vi "WildBugChilGru.vi"() -> ()   [LabVIEW 2014]
uses:
  <vilib>/Utility/miscctls.llb/LVPointTypeDef.ctl
  <vilib>/Utility/xml.llb/Write to XML File(string).vi
  <vilib>/Platform/browser.llb/Open URL in Default Browser (string).vi
  <vilib>/Instr/_visa.llb/VISA Configure Serial Port (Instr).vi
  <vilib>/Analysis/3filter.llb/IIR Filter (DBL).vi
  <vilib>/gmath/NI_Gmath.lvlib
  <vilib>/Analysis/NI_AALBase.lvlib
  <vilib>/ptbypt/NI_PtbyPt.lvlib
panel:
  in  "Autoskalierung Leistung":bool
  in  "Registerkarte 2":enum32{"Seite 1", "Seite 2"}(tab)
  in  "Autoskalierung AFR":bool
  in  "Resetskalierung AFR":bool
  out "Text Rolle":string="Dyno"
  out "Text Zündung":string="Ignition"
  in  "Resetskalierung Leistung":bool
  out "Engine\n[1/min]":cluster{dbl, dbl}(knob) scale=0.0..14000.0
  out "Untersetzung\nermittelt":bool
  out "Rear Tire\n[km/h]":dbl(knob) scale=0.0..200.0
  out "Leistungs-Graph":cluster{dbl[], dbl[]}[](graph)
  out "Untersetzung":dbl format="%.2f"
  out "Untersetzung-Graph":dbl(graph)=4.054054054054054 caption="Untersetzung"
  out "AFR,EGT-Graph":cluster{dbl[], dbl[]}[](graph)
  out "AFR":dbl min=10.0 max=20.0 format="%.1f"
  out "[°C]":dbl
  out "Y-Koord. Graph-Reset-Button (782)":i32=782
  out "Höhe Leistungs-Graph (646)":u32=646
  out "Strecke [m]":dbl=150.82399680000003
  out "dT":dbl=0.02
  out "Cyclecounter":dbl=574.0
  out "Datum+Zeit":string="24.01.2021 11:37"
  out "n(Pmax)":dbl=8917.488266666665
  out "Pmax":dbl=19.664704640664365
  out "Lauf abgebrochen":bool
  out "Auto-Datei":string
  out "Auto-Gespeichert":bool
  in  "Auto-Pfad":path
  in  "Auto-Speichern":bool
  out "n(Rolle) [1/min]":dbl=2046.0
  in  "Fahrzeugdaten":string
  out "Ergebnis":string
  out "Pmax":string="0,0 PS"
  in  "Drucken":bool
  in  "Speichern":bool
  in  "Start":bool
  in  "Ende":bool
  in  "Spenden":bool
  in  "Registerkarte":T1(tab)=enum."Mode & Recalc"
  in  "ignition [Imp/rev]":dbl=1.0 format="%#.2f"
  in  "Übersetzung ermitteln aus":T2(ring)
  in  "gear ratio [1:]":dbl=4.0 min=0.0001
  in  "tire circumferential  [m]":dbl=1.222 min=0.0001
  in  "duration  [s]":u8=5
  in  "nCrank/nDyno":dbl=4.008 format="%#.2f"
  in  "air temperature [°C]":dbl=23.2 format="%#.1g"
  in  "air pressure [mbar]":dbl=100.34 min=0.0001
  in  "Messung Klimadaten":bool=TRUE
  in  "Filter Zündsignal":bool
  in  "v min [km/h]":u16=40
  in  "moving average Mittelwert":u8=35
  in  "difference quotient":u8=12
  in  "n min [1/min]":u16=5000
  in  "torque loss M1 [Nm] @ n1":dbl min=0.0
  in  "dynospeed of torque loss. n1 [1/min]":u16=1 min=1
  in  "torque loss M0 [Nm] @ n = 0":dbl min=0.0
  in  "incr./rev. dyno  [Inkr/U]":u16=100 min=1
  in  "circum. dyno [m]":dbl=0.942 min=0.0001
  in  "Inertia dyno [kgm²]":dbl=0.164 min=0.0001
  in  "record dyno speed":bool
  in  "Lambda":bool caption="Messung Klimadaten"
  in  "AFR, EGT":bool caption="Messung Klimadaten"
  in  "Title Diagram":string
  in  "Recalc":bool
  in  "Leistung":bool=TRUE caption="Messung Klimadaten"
  in  "Logfiles":bool
  out "Datenspeicher":T3={"Fahrzeugdaten"="§$", "Auto-Pfad"="24.01.2021 11:37|", "Rolle [Inkr/U]"=100, "Rollenumfang [m]"=0.942, "Rollenträgheit [kgm²]"=0.164, "Zündung [Imp/U]"=1.0, "Getriebe [1:]"=4.0, "Reifenumfang [m] "=1.222, "element"=0.0, "Gl. Mittelwert"=35, "Differenzenquotient"=12, "AFR EGT"=0, "dT [s]"=0.02, "Strecke [m]"=150.82399680000003, "Lufttemperatur [°C]"=23.2, "Mv: n1 [1/min]"=1.0, "Luftdruck [mbar]"=100.34, "nRolle"=array[575 elements], "nWelle"=array[575 elements], "AFR"=[15.4, 15.4, 15.4, 15.4, 15.4, 15.4, 15.4, 15.4, 15.4, 15.4, 14.9, 14.9, 14.9, 14.9, 14.9, 14.9, 14.9, 14.9, 14.9, 14.9, 15.0, 15.0, 15.0, 15.0, 15.0, 15.4, 15.4, 15.4, 15.4, 15.4, 15.1, 15.1, 15.1, 15.1, 15.1, 14.9, 14.9, 14.9, 14.9, 14.9, 15.2, 15.2, 15.2, 15.2, 15.2, 15.3, 15.3, 15.3, 15.3, 15.3, 15.3, 15.3, 15.3, 15.3, 15.3, 15.0, 15.0, 15.0, 15.0, 15.0, 14.9, 14.9, 14.9, 14.9, 14.9, 15.2, 15.2, 15.2, 15.2, 15.2, 15.4, 15.4, 15.4, 15.4, 15.4, 14.9, 14.9, 14.9, 14.9, 14.9, 14.9, 14.9, 14.9, 14.9, 14.9, 15.1, 15.1, 15.1, 15.1, 15.1, 15.3, 15.3, 15.3, 15.3, 15.3, 15.2, 15.2, 15.2, 15.2, 15.2, 15.0, 15.0, 15.0, 15.0, 15.0, 15.3, 15.3, 15.3, 15.3, 15.3, 15.1, 15.1, 15.1, 15.1, 15.1, 15.3, 15.3, 15.3, 15.3, 15.3, 15.0, 15.0, 15.0, 15.0, 15.0, 15.0, 15.0, 15.0, 15.0, 15.0, 15.3, 15.3, 15.3, 15.3, 15.3, 15.2, 15.2, 15.2, 15.2, 15.2, 15.2, 15.2, 15.2, 15.2, 15.2, 15.0, 15.0, 15.0, 15.0, 15.0, 15.2, 15.2, 15.2, 15.2, 15.2, 15.4, 15.4, 15.4, 15.4, 15.4, 15.2, 15.2, 15.2, 15.2, 15.2, 15.1, 15.1, 15.1, 15.1, 15.1, 15.3, 15.3, 15.3, 15.3, 15.3, 15.3, 15.3, 15.3, 15.3, 15.3, 14.9, 14.9, 14.9, 14.9, 14.9, 15.3, 15.3, 15.3, 15.3, 15.3, 15.0, 15.0, 15.0, 15.0, 15.0, 15.3, 15.3, 15.3, 15.3, 15.3, 15.3, 15.3, 15.3, 15.3, 15.3, 15.2, 15.2, 15.2, 15.2, 15.2, 15.0, 15.0, 15.0, 15.0, 15.0, 15.0, 15.0, 15.0, 15.0, 15.0, 15.2, 15.2, 15.2, 15.2, 15.2, 15.2, 15.2, 15.2, 15.2, 15.2, 15.4, 15.4, 15.4, 15.4, 15.4, 15.0, 15.0, 15.0, 15.0, 15.0, 15.1, 15.1, 15.1, 15.1, 15.1, 15.0, 15.0, 15.0, 15.0, 15.0, 15.1, 15.1, 15.1, 15.1, 15.1, 15.1, 15.1, 15.1, 15.1, 15.1, 15.4, 15.4, 15.4, 15.4, 15.4, 15.0, 15.0, 15.0, 15.0, 15.0, 15.2, 15.2, 15.2, 15.2, 15.2, 15.0, 15.0, 15.0, 15.0, 15.0, 15.0, 15.0, 15.0, 15.0, 15.0, 15.3, 15.3, 15.3, 15.3, 15.3, 14.9, 14.9, 14.9, 14.9, 14.9, 15.2, 15.2, 15.2, 15.2, 15.2, 15.1, 15.1, 15.1, 15.1, 15.1, 15.2, 15.2, 15.2, 15.2, 15.2, 15.0, 15.0, 15.0, 15.0, 15.0, 15.4, 15.4, 15.4, 15.4, 15.4, 15.0, 15.0, 15.0, 15.0, 15.0, 15.4, 15.4, 15.4, 15.4, 15.4, 15.1, 15.1, 15.1, 15.1, 15.1, 15.3, 15.3, 15.3, 15.3, 15.3, 15.0, 15.0, 15.0, 15.0, 15.0, 14.9, 14.9, 14.9, 14.9, 14.9, 15.1, 15.1, 15.1, 15.1, 15.1, 15.1, 15.1, 15.1, 15.1, 15.1, 15.0, 15.0, 15.0, 15.0, 15.0, 15.2, 15.2, 15.2, 15.2, 15.2, 15.4, 15.4, 15.4, 15.4, 15.4, 15.2, 15.2, 15.2, 15.2, 15.2, 15.2, 15.2, 15.2, 15.2, 15.2, 14.9, 14.9, 14.9, 14.9, 14.9, 15.0, 15.0, 15.0, 15.0, 15.0, 15.2, 15.2, 15.2, 15.2, 15.2, 14.9, 14.9, 14.9, 14.9, 14.9, 15.1, 15.1, 15.1, 15.1, 15.1, 15.2, 15.2, 15.2, 15.2, 15.2, 15.0, 15.0, 15.0, 15.0, 15.0, 15.0, 15.0, 15.0, 15.0, 15.0, 15.2, 15.2, 15.2, 15.2, 15.2, 15.3, 15.3, 15.3, 15.3, 15.3, 15.0, 15.0, 15.0, 15.0, 15.0, 15.0, 15.0, 15.0, 15.0, 15.0, 15.1, 15.1, 15.1, 15.1, 15.1, 15.3, 15.3, 15.3, 15.3, 15.3, 15.1, 15.1, 15.1, 15.1, 15.1, 15.3, 15.3, 15.3, 15.3, 15.3, 15.1, 15.1, 15.1, 15.1, 15.1, 15.0, 15.0, 15.0, 15.0, 15.0, 15.2, 15.2, 15.2, 15.2, 15.2, 14.9, 14.9, 14.9, 14.9, 14.9, 15.3, 15.3, 15.3, 15.3, 15.3, 15.1, 15.1, 15.1, 15.1, 15.1, 15.4, 15.4, 15.4, 15.4, 15.4, 15.4, 15.4, 15.4, 15.4, 15.4, 15.4, 15.4, 15.4, 15.4, 15.4, 14.9, 14.9, 14.9, 14.9, 14.9, 15.2, 15.2, 15.2, 15.2, 15.2, 15.0, 15.0, 15.0, 15.0, 15.0, 15.0, 15.0, 15.0, 15.0, 15.0, 15.4, 15.4, 15.4, 15.4, 15.4, 15.4, 15.4, 15.4, 15.4, 15.4, 15.4, 15.4, 15.4, 15.4, 15.4, 15.1, 15.1, 15.1, 15.1, 15.1, 15.2, 15.2, 15.2, 15.2, 15.2, 15.2, 15.2, 15.2, 15.2, 15.2, 15.1, 15.1, 15.1, 15.1, 15.1, 15.2, 15.2, 15.2, 15.2, 15.2, 15.3, 15.3, 15.3, 15.3, 15.3], "EGT"=array[575 elements], "Übersetzung ermitteln aus"=0, "[s]"=5.0, "Mv: M0 [Nm]"=0.0, "Mv: M1 [Nm]"=0.0, "n vom Gas [1/min]"=5000.0, "dT-Array [s]"=array[575 elements], [], "Boolesch"=TRUE, "Serielle Schnittstelle"="COM6", "nKuWe/nRolle"=4.008, "v vom Gas [km/h]"=40.0}
  out "COM-Fehlerrate":string="0 / 0,0%"
  in  "Konfiguration:":bool
  out "Füllstand Lesepuffer":u64(slide)=1 scale=1.0..100.0
  out "Lesepuffer":string="\r\n"
  in  "Serielle Schnittstelle":refnum<visa-resource-name>="COM6"
  # "Power measurement:\n1. constant speed\n2. START [F1]\n3. hold speed\n4. @ GO: open throttle\n5. release gas"
  # "WildBugGruChil Dyno v3.0.1"
  # "ratio engine/dyno"
  # "manual <> measure"
  # "Dashboard <> Measure"
  # "AFR / l &  EGT"
  # "AFR <> l"
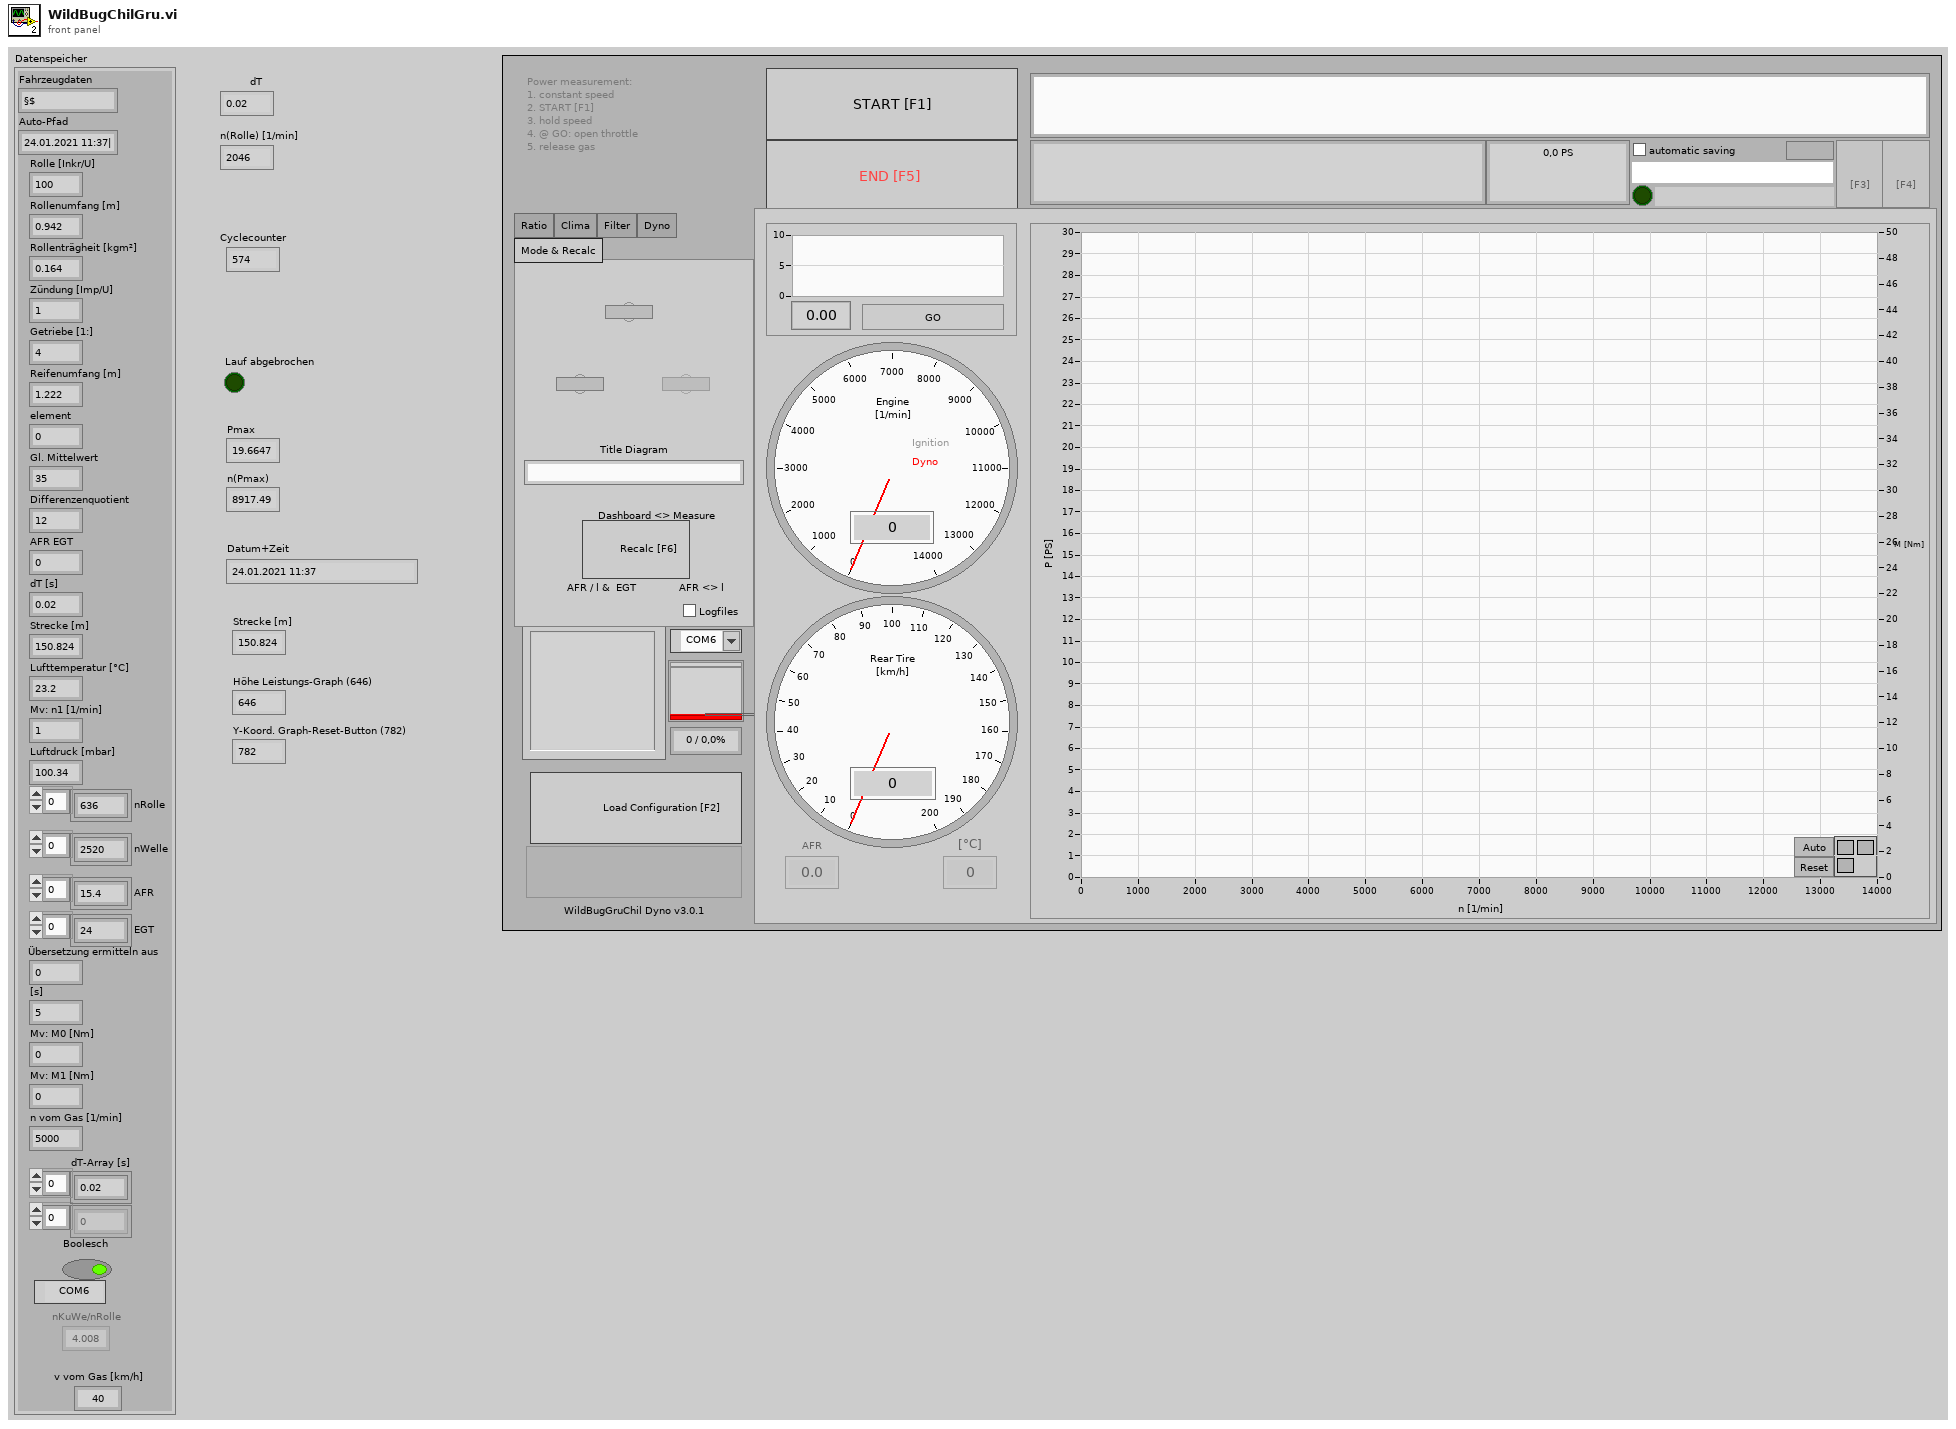
[diagram p1: front panel]
types:
  T1 = enum32{"Ratio", "Clima", "Filter", "Dyno", "Mode & Recalc"}
  T2 = enum8{"ignition signal", "gear ratio & speed", "nCrank / nDyno", "vario (km/h)"}
  T3 = cluster{"Fahrzeugdaten":string, "Auto-Pfad":string, "Rolle [Inkr/U]":u16, "Rollenumfang [m]":dbl, "Rollenträgheit [kgm²]":dbl, "Zündung [Imp/U]":dbl, "Getriebe [1:]":dbl, "Reifenumfang [m] ":dbl, "element":dbl, "Gl. Mittelwert":u8, "Differenzenquotient":u8, "AFR EGT":u8, "dT [s]":dbl, "Strecke [m]":dbl, "Lufttemperatur [°C]":dbl, "Mv: n1 [1/min]":dbl, "Luftdruck [mbar]":dbl, "nRolle":dbl[], "nWelle":dbl[], "AFR":dbl[], "EGT":dbl[], "Übersetzung ermitteln aus":u8, "[s]":dbl, "Mv: M0 [Nm]":dbl, "Mv: M1 [Nm]":dbl, "n vom Gas [1/min]":dbl, "dT-Array [s]":dbl[], i32[], "Boolesch":bool, "Serielle Schnittstelle":refnum<visa-resource-name>, "nKuWe/nRolle":dbl, "v vom Gas [km/h]":dbl}
  T4 = enum8{"Enabled", "Disabled", "Disabled and Grayed Out"}
  T5 = cluster{"Fahrzeugdaten":string, "Auto-Pfad":string, "Rolle [Inkr/U]":u16, "Rollenumfang [m]":dbl, "Rollenträgheit [kgm²]":dbl, "Zündung [Imp/U]":dbl, "Getriebe [1:]":dbl, "Reifenumfang [m] ":dbl, "element":dbl, "Gl. Mittelwert":u8, "Differenzenquotient":u8, u8, "dT [s]":dbl, "Strecke [m]":dbl, "Lufttemperatur [°C]":dbl, "Mv: n1 [1/min]":dbl, "Luftdruck [mbar]":dbl, "nRolle":dbl[], "nWelle":dbl[], "AFR":dbl[], "EGT":dbl[], "Übersetzung ermitteln aus":u8, "[s]":dbl, "Mv: M0 [Nm]":dbl, "Mv: M1 [Nm]":dbl, "n vom Gas [1/min]":dbl, "dT-Array [s]":dbl[], i32[], "Boolesch":bool, "Serielle Schnittstelle":refnum<visa-resource-name>, "nKuWe/nRolle":dbl, "v vom Gas [km/h]":dbl}
  T6 = enum32{"invalid app kind", "Development System", "Run Time System", "Student Edition", "Embedded LabVIEW", "Evaluation", "Custom"}
  T7 = cluster{string, string, "incr./rev. dyno  [Inkr/U]":u16, "circum. dyno [m]":dbl, "Inertia dyno [kgm²]":dbl, "ignition [Imp/rev]":dbl, "gear ratio [1:]":dbl, "tire circumferential  [m] ":dbl, "mean value":dbl, "moving average Mittelwert":u8, "difference quotient ":u8, u32, dbl, "Strecke [m]":dbl, "air temperature [°C]":dbl, "dynospeed of torque loss. n1 [1/min]":u16, "air pressure [mbar]":dbl, dbl[], dbl[], dbl[], dbl[], "Übersetzung ermitteln aus":enum8{"ignition signal", "gear ratio & speed", "nCrank / nDyno", "vario (km/h)"}, "duration  [s]":u8, "torque loss M0 [Nm] @ n = 0 ":dbl, "torque loss M1 [Nm] @ n1":dbl, "n min [1/min]":u16, dbl[], i32[], "Messung Klimadaten":bool, "VISA-Referenz (Ausgang)":refnum<visa-resource-name>, "nCrank/nDyno":dbl, "v min [km/h]":u16}
  T8 = typedef "LVPointTypeDef.ctl" = cluster{"Horizontal":i16, "Vertical":i16}
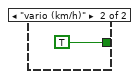
[diagram p3: hidden frame]
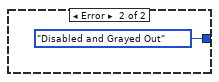
[diagram p5: hidden frame]
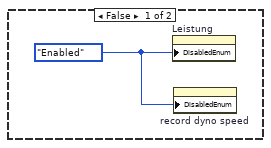
[diagram p6: hidden frame]
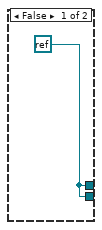
[diagram p7: hidden frame]
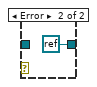
[diagram p8: hidden frame]
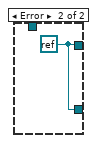
[diagram p9: hidden frame]
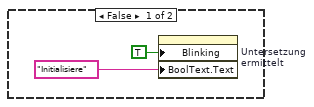
[diagram p10: hidden frame]
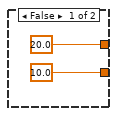
[diagram p11: hidden frame]
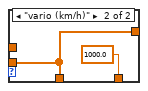
[diagram p20: hidden frame]
diagram:
  w3 = FALSE
  n1 = while {
    stop <- w9 stop-if-true
    n2 = event shown="[6] \"Spenden\": Wertänderung" {
      selector: _ -> [_ _ _ _ _ _ _ _ _ _ _ _ _ _ _ _ _ _]
      dyn-events: _ -> [_ _ _ _ _ _ _ _ _ _ _ _ _ _ _ _ _ _]
      timeout: _ -> [_ _ _ _ _ _ _ _ _ _ _ _ _ _ _ _ _ _]
      tunnel: [_ _ _ TRUE _ _ _ _ _ _ _ _ _ _ _ _ _ _] -> w9
      event "Konfiguration:": Value Change {
        n3 = event-data() -> ("OldVal"=w11:bool)  [unwired: 1 in, 5 out]
        n4 = flat-sequence {
          tunnel: [w55] -> w12
          tunnel: w11 -> [w55]
          tunnel: w12 -> [w56]
          frame #0 {
            n5 = property on="Datenspeicher" class="Cluster (strikt)"() -> ("Value"=w54:T3)  [unwired: 2 in, 2 out]
            n6 = call "LoadCluster (SubVI).vi"("Datenspeicher"=w54) -> ("Value"=w53:T5)  [unwired: 8 in, 2 out]
            n7 = Unbundle(w53) -> ("Fahrzeugdaten"=w20:string, "Auto-Pfad"=w28:string, "Rolle [Inkr/U]"=w52:u16, "Rollenumfang [m]"=w51:dbl, "Rollenträgheit [kgm²]"=w50:dbl, "Zündung [Imp/U]"=w49:dbl, "Getriebe [1:]"=w48:dbl, "Reifenumfang [m]"=w47:dbl, "Gl. Mittelwert"=w46:u8, "Differenzenquotient"=w45:u8, w15:u8, "Lufttemperatur [°C]"=w44:dbl, "Mv: n1 [1/min]"=w25:dbl, "Luftdruck [mbar]"=w43:dbl, "Übersetzung ermitteln aus"=w40:u8, "[s]"=w42:dbl, "Mv: M0 [Nm]"=w36:dbl, "Mv: M1 [Nm]"=w35:dbl, "n vom Gas [1/min]"=w41:dbl, "Boolesch"=w39:bool, "nKuWe/nRolle"=w38:dbl, "v vom Gas [km/h]"=w37:dbl)  [unwired: 10 out]
            n8 = property on="duration  [s]" class="DigWert (strikt)"("Value"=w42) -> ()  [unwired: 2 in, 2 out]
            n9 = property on="Übersetzung ermitteln aus" class="Enum (strikt)"("Val(Sgnl)"=w40) -> ()  [unwired: 2 in, 2 out]
            n10 = property on="incr./rev. dyno  [Inkr/U]" class="DigWert (strikt)"("Value"=w52) -> ()  [unwired: 2 in, 2 out]
            n11 = property on="circum. dyno [m]" class="DigWert (strikt)"("Value"=w51) -> ()  [unwired: 2 in, 2 out]
            n12 = property on="Inertia dyno [kgm²]" class="DigWert (strikt)"("Value"=w50) -> ()  [unwired: 2 in, 2 out]
            n13 = property on="ignition [Imp/rev]" class="DigWert (strikt)"("Value"=w49) -> ()  [unwired: 2 in, 2 out]
            n14 = property on="gear ratio [1:]" class="DigWert (strikt)"("Value"=w48) -> ()  [unwired: 2 in, 2 out]
            n15 = property on="tire circumferential  [m]" class="DigWert (strikt)"("Value"=w47) -> ()  [unwired: 2 in, 2 out]
            n16 = property on="moving average Mittelwert" class="DigWert (strikt)"("Value"=w46) -> ()  [unwired: 2 in, 2 out]
            n17 = property on="difference quotient" class="DigWert (strikt)"("Value"=w45) -> ()  [unwired: 2 in, 2 out]
            n18 = property on="air temperature [°C]" class="DigWert (strikt)"("Value"=w44) -> ()  [unwired: 2 in, 2 out]
            n19 = property on="air pressure [mbar]" class="DigWert (strikt)"("Value"=w43) -> ()  [unwired: 2 in, 2 out]
            n20 = property on="n min [1/min]" class="DigWert (strikt)"("Value"=w41) -> ()  [unwired: 2 in, 2 out]
            n21 = property on="Messung Klimadaten" class="Bool. (strikt)"("Val(Sgnl)"=w39) -> ()  [unwired: 2 in, 2 out]
            n22 = property on="nCrank/nDyno" class="DigWert (strikt)"("Value"=w38) -> ()  [unwired: 2 in, 2 out]
            n23 = property on="v min [km/h]" class="DigWert (strikt)"("Value"=w37) -> ()  [unwired: 2 in, 2 out]
            n24 = Number To Boolean Array(number=w15) -> (Boolean array=w17:bool[])
            n25 = property on="torque loss M1 [Nm] @ n1" class="DigWert (strikt)"("Value"=w35) -> ()  [unwired: 2 in, 2 out]
            n26 = property on="torque loss M0 [Nm] @ n = 0" class="DigWert (strikt)"("Value"=w36) -> ()  [unwired: 2 in, 2 out]
            n27 = Index Array(array=w17, index=0) -> (element=w14:bool)
            n28 = Index Array(array=w17, index=1) -> (element=w13:bool)
            n29 = property on="Lambda" class="Bool. (strikt)"("Val(Sgnl)"=w13) -> ()  [unwired: 2 in, 2 out]
            n30 = property on="AFR, EGT" class="Bool. (strikt)"("Value"=w14) -> ()  [unwired: 2 in, 2 out]
            n31 = Search/Split String "führende Fahrzeugdaten wegschneiden"(string=w20, search string/char (-)="§$") -> (substring before match=w19:string, match + rest of string=w22:string)  [unwired: 1 in, 1 out]
            n32 = Search/Split String "führendes Datum+Zeit wegschneiden"(string=w28, search string/char (-)="|") -> (substring before match=w29:string, match + rest of string=w32:string)  [unwired: 1 in, 1 out]
            n33 = Max & Min(x=1, y=w25) -> (max(x,y)=w27:dbl)  [unwired: 1 out]
            n34 = String Subset(string=w22, offset (0)=2) -> (substring=w21:string)  [unwired: 1 in]
            n35 = String Subset(string=w32, offset (0)=1) -> (substring=w30:string)  [unwired: 1 in]
            n36 = String To Path(string=w30) -> (path=w34:path)
            n37 = property on="dynospeed of torque loss. n1 [1/min]" class="DigWert (strikt)"("Value"=w27) -> ()  [unwired: 2 in, 2 out]
            n38 = property on="Title Diagram" class="Str"("Value"=w21) -> ()  [unwired: 2 in, 2 out]
            n39 = property on="Datum+Zeit" class="Str"("Value"=w29) -> ()  [unwired: 2 in, 2 out]
            n40 = property on="Fahrzeugdaten" class="Str"("Value"=w19) -> ()  [unwired: 2 in, 2 out]
            n41 = property on="Auto-Pfad" class="Pfad"("Value"=w34) -> ()  [unwired: 2 in, 2 out]
          }
          frame #1 {
            n42 = property on="Konfiguration:" class="Bool. (strikt)"("Value"=w56) -> ()  [unwired: 2 in, 2 out]
          }
        }
      }
      event "Drucken": Value Change {
        n43 = event-data() -> ("OldVal"=w57:bool)  [unwired: 1 in, 5 out]
        n44 = flat-sequence {
          tunnel: [w65] -> w58
          tunnel: w57 -> [w65]
          tunnel: w58 -> [w66]
          frame #0 {
            n45 = control-ref of="Fahrzeugdaten"() -> (w63:refnum<vi>)
            n46 = control-ref of="Ergebnis"() -> (w62:refnum<vi>)
            n47 = control-ref of="Title Diagram"() -> (w61:refnum<vi>)
            n48 = control-ref of="Leistungs-Graph"() -> (w64:refnum<vi>)
            n49 = control-ref of="AFR,EGT-Graph"() -> (w60:refnum<vi>)
            n50 = local read "AFR, EGT"() -> (w59:bool)
            n51 = call "PrintGraph (SubVI).vi"("AFR,EGT-Graph Ref"=w60, "AFR, EGT"=w59, "Überschrift"=w61, "Ergebnis"=w62, "Fahrzeugdaten"=w63, "P+M Graph Ref"=w64) -> ()  [unwired: 6 in]
          }
          frame #1 {
            n52 = property on="Drucken" class="Bool. (strikt)"("Value"=w66) -> ()  [unwired: 2 in, 2 out]
          }
        }
      }
      event "Speichern": Value Change {
        n53 = event-data() -> ("OldVal"=w67:bool)  [unwired: 1 in, 5 out]
        n54 = flat-sequence {
          frame #0 {
            n55 = property on="Auto-Gespeichert" class="Bool. (strikt)"("Value"=FALSE) -> ()  [unwired: 2 in, 2 out]
            n56 = property on="Auto-Datei" class="Str"("Value"="") -> ()  [unwired: 2 in, 2 out]
          }
          frame #1 {
            n57 = local read "Auto-Pfad"() -> (w79:path)
            n58 = property on="Auto-Speichern" class="Bool. (strikt)"() -> ("Value"=w73:bool)  [unwired: 2 in, 2 out]
            n59 = call <vilib>:"Check if File or Folder Exists.vi"("path"=w79) -> ("file or folder exists?"=w78:bool, "dup path"=w75:path)  [unwired: 8 in, 1 out]
            n60 = Not(x=w78) -> (.not. x?=w77:bool)
            n61 = And(x=w73, y=w77) -> (x .and. y?=w76:bool)
            n62 = And(x=w73, y=w78) -> (x .and. y?=w70:bool)
            n63 = call "Meldung an Benutzer2"("Enable"=w76) -> ()  [unwired: 9 in, 2 out]
            n64 = case shown="True" w70 {
              tunnel: [path "" w95] -> w80
              tunnel: w75 -> [_ w94]
              tunnel: ["" w88] -> w71
              frame False {
              }
              frame True {
                n65 = Get Date/Time In Seconds() -> (seconds since 1Jan1904=w98:timestamp)
                n66 = local read "Pmax"() -> (w91:dbl)
                n67 = local read "n(Pmax)"() -> (w90:dbl)
                n68 = Path To String(path=w94) -> (string=w97:string)
                n69 = Format Into String(format string="%,; %.1f_%d.xml" ("Format-String"), w91, w90) -> (resulting string=w86:string)  [unwired: 2 in, 1 out]
                n70 = Format Date/Time String(time format string (%c)="%y%m%d_%H%M%S_", seconds (now)=w98) -> (date/time string=w87:string)  [unwired: 1 in]
                n71 = Concatenate Strings(w97, "\\", w87, w86) -> (w96:string)
                n72 = Concatenate Strings(w87, w86) -> (w88:string)
                n73 = String To Path(string=w96) -> (path=w95:path)
              }
            }
            n74 = control-ref of="Datenspeicher"() -> (w81:refnum<vi>)
            n75 = call "SaveCluster (SubVI).vi"("selected path"=w80, "Datenspeicher 2"=w81) -> ("Kein Fehler"=w74:bool)
            n76 = And(x=w70, y=w74) -> (x .and. y?=w72:bool)
            n77 = case shown="True" w72 {
              tunnel: w71 -> [_ w83]
              frame False {
              }
              frame True {
                n78 = property on="Auto-Gespeichert" class="Bool. (strikt)"("Value"=TRUE) -> ()  [unwired: 2 in, 2 out]
                n79 = property on="Auto-Datei" class="Str"("Value"=w83) -> ()  [unwired: 2 in, 2 out]
              }
            }
          }
        }
        n80 = local write "Speichern"(w67) -> ()
      }
      event "Ende": Value Change {
        w108 = 0.0 ("element")
        n81 = event-data() -> ("OldVal"=w106:bool)  [unwired: 1 in, 5 out]
        n82 = local read "Datenspeicher"() -> (w109:T3)
        n83 = flat-sequence {
          tunnel: [w138] -> w105
          tunnel: w106 -> [w138]
          frame #0 {
            n84 = Wait (ms)(milliseconds to wait=u32 200) -> ()  [unwired: 1 out]
          }
        }
        n85 = Unbundle By Name(w109) -> ("Auto-Pfad"=w100:string, "Rolle [Inkr/U]"=w130:u16, "Rollenumfang [m]"=w129:dbl, "Rollenträgheit [kgm²]"=w128:dbl, "Zündung [Imp/U]"=w127:dbl, "Getriebe [1:]"=w126:dbl, "Reifenumfang [m]"=w125:dbl, "Gl. Mittelwert"=w124:u8, "Differenzenquotient"=w123:u8, "Fahrzeugdaten"=w122:string, "Lufttemperatur [°C]"=w121:dbl, "Mv: n1 [1/min]"=w120:dbl, "Luftdruck [mbar]"=w118:dbl, "nRolle"=w119:dbl[], "Übersetzung ermitteln aus"=w117:u8, "[s]"=w116:dbl, "Mv: M0 [Nm]"=w115:dbl, "Mv: M1 [Nm]"=w114:dbl, "n vom Gas [1/min]"=w113:dbl, "Boolesch"=w112:bool, "Serielle Schnittstelle"=w107:refnum<visa-resource-name>, "nWelle"=w104:dbl[], "AFR"=w102:dbl[], "EGT"=w101:dbl[], "v vom Gas [km/h]"=w103:dbl, "AFR EGT"=w99:u8)  [unwired: 3 out]
        n86 = call <vilib>:"Application Directory.vi"() -> ("Application Directory"=w133:path)
        n87 = local write "Ende"(w105) -> ()
        n88 = Bundle By Name(cluster=w109, "Auto-Pfad"=w100, "Rolle [Inkr/U]"=w130, "Rollenumfang [m]"=w129, "Rollenträgheit [kgm²]"=w128, "Zündung [Imp/U]"=w127, "Getriebe [1:]"=w126, "Reifenumfang [m]"=w125, "element"=0.0, "Gl. Mittelwert"=w124, "Differenzenquotient"=w123, "Fahrzeugdaten"=w122, "element"=w108, "element"=w108, "Lufttemperatur [°C]"=w121, "Mv: n1 [1/min]"=w120, "Luftdruck [mbar]"=w118, "nRolle"=w119, "Übersetzung ermitteln aus"=w117, "[s]"=w116, "Mv: M0 [Nm]"=w115, "Mv: M1 [Nm]"=w114, "n vom Gas [1/min]"=w113, "Boolesch"=w112, "Serielle Schnittstelle"=w107, "nWelle"=w104, "AFR"=w102, "EGT"=w101, "v vom Gas [km/h]"=w103, "AFR EGT"=w99) -> (w110:T3)
        n89 = Build Path(base path=w133, name or relative path="Konfig.xml") -> (appended path=w131:path)
        n90 = Flatten To XML(anything=w110) -> (xml string=w135:string)
        n91 = call-poly <vilib>:"Write to XML File.vi"("XML Input"=w135, "XML File Path"=w131) -> ("error out"=w134:errorcluster)  [unwired: 7 in, 2 out]
        n92 = case shown="Kein Fehler" w134 {
          frame No Error {
          }
          frame Error {
          }
        }
      }
      event "Serielle Schnittstelle": Value Change {
        n93 = event-data() -> ()  [unwired: 1 in, 6 out]
        n94 = property on="Start" class="Bool. (strikt)"("DisabledEnum"=T4."Enabled" ("Deaktiviert")) -> ()  [unwired: 2 in, 2 out]
      }
      event "Messung Klimadaten": Value Change {
        n95 = event-data() -> ("NewVal"=w140:bool)  [unwired: 1 in, 5 out]
        n96 = case shown="True" w140 {
          frame True {
            w141 = T4."Disabled and Grayed Out" ("Deaktiviert")
            n97 = property on="air temperature [°C]" class="DigWert (strikt)"("DisabledEnum"=w141) -> ()  [unwired: 2 in, 2 out]
            n98 = property on="air pressure [mbar]" class="DigWert (strikt)"("DisabledEnum"=w141) -> ()  [unwired: 2 in, 2 out]
          }
          frame False {
            w142 = T4."Enabled" ("Deaktiviert")
            n99 = property on="air temperature [°C]" class="DigWert (strikt)"("DisabledEnum"=w142) -> ()  [unwired: 2 in, 2 out]
            n100 = property on="air pressure [mbar]" class="DigWert (strikt)"("DisabledEnum"=w142) -> ()  [unwired: 2 in, 2 out]
          }
        }
      }
      event "Spenden": Value Change {
        n101 = event-data() -> ()  [unwired: 1 in, 6 out]
        n102 = case shown="True" "Spenden" {
          frame False {
          }
          frame True {
            (unwired) "https://www.paypal.com/cgi-bin/webscr?cmd=_s-xclick&hosted_button_id=5HCL4L3EEXS64&source=url"  # Spende an august.gruendl@gmx.at
            w144 = "https://www.paypal.com/cgi-bin/webscr?cmd=_s-xclick&hosted_button_id=8SA7Y5J5P5N3W&source=url"  # Spende an WildBugChilGru@gmx.net
            n103 = call-poly <vilib>:"Open URL in Default Browser.vi"("URL"=w144) -> ()  [unwired: 5 in, 2 out]
          }
        }
      }
      event "Recalc": Value Change {
        n104 = event-data() -> ("OldVal"=w147:bool)  [unwired: 1 in, 5 out]
        n105 = property on="Recalc" class="Bool. (strikt)"("Value"=w147) -> ()  [unwired: 2 in, 2 out]
        n106 = property on="Datenspeicher" class="Cluster (strikt)"() -> ("Value"=w145:T3)  [unwired: 2 in, 2 out]
        n107 = call "ReCalc.vi"("Berechnen"=TRUE, "Datenspeicher"=w145) -> ()  [unwired: 3 in]
      }
      event "Übersetzung ermitteln aus": Value Change {
        w151 = 2
        w157 = 1
        n108 = event-data() -> ("NewVal"=w175:T2)  [unwired: 1 in, 5 out]
        n109 = case shown="\"vario (km/h)\"" w175 {
          tunnel: [w191 w192 w194 w197] -> w176
          tunnel: [w191 w193 w194 w196] -> w173
          tunnel: [w191 w192 w195 w196] -> w165
          tunnel: [w191 w193 w195 w197] -> w172
          tunnel: [T4."Enabled" ("Deaktiviert") w192 w194 w196] -> w171
          frame "vario (km/h)" {
            w191 = T4."Disabled and Grayed Out" ("Deaktiviert")
          }
          frame "nCrank / nDyno" {
            w193 = T4."Enabled" ("Deaktiviert")
            w192 = T4."Disabled and Grayed Out" ("Deaktiviert")
          }
          frame "ignition signal", Default {
            w195 = T4."Enabled" ("Deaktiviert")
            w194 = T4."Disabled and Grayed Out" ("Deaktiviert")
          }
          frame "gear ratio & speed" {
            w196 = T4."Disabled and Grayed Out" ("Deaktiviert")
            w197 = T4."Enabled" ("Deaktiviert")
          }
        }
        n110 = case shown="\"vario (km/h)\"" w175 {
          tunnel: ["n [1/min]" "M [Nm]"] -> w174
          tunnel: [200.0 14000.0] -> w164
          tunnel: ["v [km/h]" "n [1/min]"] -> w149
          tunnel: [14000.0 50.0] -> w170
          tunnel: [u32 16777216 w185] -> w168
          tunnel: [u32 16711680 w185] -> w167
          tunnel: [FALSE TRUE] -> w166
          frame "vario (km/h)" {
          }
          frame Default {
            w185 = u32 9868950
          }
        }
        n111 = property on="Leistungs-Graph" class="XYGraph (strikt)"("ActYScl"=w157, "YScale.NameLbl.Text"=w174, "YScale.Maximum"=w170, "XScale.NameLbl.Text"=w149, "XScale.Maximum"=w164) -> ("Height"=w163:u32, "YScale.NameLbl.Width"=w162:u32, "Top"=w159:i32, "Width"=w154:u32, "XScale.NameLbl.Width"=w153:u32, "Left"=w152:i32)  [unwired: 2 in, 2 out]
        n112 = property on="Text Zündung" class="Str"("Text.TextColor"=w167) -> ()  [unwired: 2 in, 2 out]
        n113 = property on="Welle [1/min]" class="Drehknopf (strikt)"("Active Slider"=1, "FG Color"=w168) -> ()  [unwired: 2 in, 2 out]
        n114 = property on="Text Rolle" class="Str"("Visible"=w166) -> ()  [unwired: 2 in, 2 out]
        n115 = Subtract(x=w154, y=w153) -> (x-y=w155:u32)
        n116 = Subtract(x=w163, y=w162) -> (x-y=w161:u32)
        n117 = Divide(x=w155, y=w151) -> (x/y=w156:dbl)
        n118 = Divide(x=w161, y=w151) -> (x/y=w160:dbl)
        n119 = Add(x=w156, y=w152) -> (x+y=w150:dbl)
        n120 = Add(x=w160, y=w159) -> (x+y=w158:dbl)
        n121 = property on="Leistungs-Graph" class="XYGraph (strikt)"("ActYScl"=w157, "YScale.NameLbl.Top"=w158, "XScale.NameLbl.Left"=w150) -> ()  [unwired: 2 in, 2 out]
        n122 = property on="AFR,EGT-Graph" class="XYGraph (strikt)"("XScale.Maximum"=w164, "XScale.NameLbl.Text"=w149, "XScale.NameLbl.Left"=w150) -> ()  [unwired: 2 in, 2 out]
        n123 = property on="nCrank/nDyno" class="DigWert (strikt)"("DisabledEnum"=w173) -> ()  [unwired: 2 in, 2 out]
        n124 = property on="v min [km/h]" class="DigWert (strikt)"("DisabledEnum"=w171) -> ()  [unwired: 2 in, 2 out]
        n125 = property on="n min [1/min]" class="DigWert (strikt)"("DisabledEnum"=w172) -> ()  [unwired: 2 in, 2 out]
        n126 = property on="gear ratio [1:]" class="DigWert (strikt)"("DisabledEnum"=w176) -> ()  [unwired: 2 in, 2 out]
        n127 = property on="tire circumferential  [m]" class="DigWert (strikt)"("DisabledEnum"=w176) -> ()  [unwired: 2 in, 2 out]
        n128 = property on="ignition [Imp/rev]" class="DigWert (strikt)"("DisabledEnum"=w165) -> ()  [unwired: 2 in, 2 out]
        n129 = property on="duration  [s]" class="DigWert (strikt)"("DisabledEnum"=w165) -> ()  [unwired: 2 in, 2 out]
        n130 = property on="Filter Zündsignal" class="Bool. (strikt)"("DisabledEnum"=w165) -> ()  [unwired: 2 in, 2 out]
        n131 = property on="Leistungs-Graph" class="XYGraph (strikt)"() -> ("Width"=w148:u32)  [unwired: 2 in, 2 out]
        n132 = property on="AFR,EGT-Graph" class="XYGraph (strikt)"("Width"=w148) -> ()  [unwired: 2 in, 2 out]
      }
      event "Resetskalierung Leistung": Value Change {
        w199 = 0.0
        n133 = event-data() -> ()  [unwired: 1 in, 6 out]
        n134 = local read "Übersetzung ermitteln aus"() -> (w202:T2)
        n135 = case shown="\"vario (km/h)\"" w202 {
          tunnel: [14000.0 200.0] -> w200
          tunnel: [50.0 14000.0] -> w201
          frame Default {
          }
          frame "vario (km/h)" {
          }
        }
        n136 = property on="Leistungs-Graph" class="XYGraph (strikt)"("XScale.Maximum"=w200, "XScale.Minimum"=w199, "ActYScl"=w199, "YScale.Maximum"=30.0, "YScale.Minimum"=w199, "ActYScl"=1, "YScale.Maximum"=w201, "YScale.Minimum"=w199) -> ()  [unwired: 2 in, 2 out]
        n137 = property on="AFR,EGT-Graph" class="XYGraph (strikt)"("XScale.Maximum"=w200, "XScale.Minimum"=w199) -> ()  [unwired: 2 in, 2 out]
      }
      event "Auto-Speichern": Value Change {
        n138 = event-data() -> ("NewVal"=w208:bool)  [unwired: 1 in, 5 out]
        n139 = case shown="True" w208 {
          frame False {
          }
          frame True {
            n140 = local read "Auto-Pfad"() -> (w211:path)
            n141 = call <vilib>:"Check if File or Folder Exists.vi"("path"=w211) -> ("file or folder exists?"=w209:bool)  [unwired: 8 in, 2 out]
            n142 = Not(x=w209) -> (.not. x?=w210:bool)
            n143 = call "Meldung an Benutzer"("Enable"=w210) -> ()  [unwired: 9 in, 2 out]
            n144 = local write "Auto-Speichern"(w209) -> ()
          }
        }
      }
      event "Fahrzeugdaten": Value Change {
        # "Fahrzeugdaten auf 3 Zeilen begrenzen\n(Recalc ist nur auf max. 3 Zeilen ausgelegt)"
        n145 = event-data() -> ("OldVal"=w214:string, "NewVal"=w215:string)  [unwired: 1 in, 4 out]
        n146 = Spreadsheet String To Array(delimiter (Tab)="\n", format string="%s", spreadsheet string=w215, array type (2D Dbl)=string[] []) -> (array=w217:string[])
        n147 = Array Size "Zeilenanzahl"(array=w217) -> (size(s)=w216:i32)
        n148 = Greater?(x=w216, y=3) -> (0:w213:bool)
        n149 = case shown="True" w213 {
          tunnel: w214 -> [_ w221]
          frame False {
          }
          frame True {
            n150 = flat-sequence {
              tunnel: w221 -> [w223]
              frame #0 {
                n151 = call "Meldung an Benutzer3"("Enable"=TRUE) -> ()  [unwired: 9 in, 2 out]
              }
              frame #1 {
                n152 = property on="Fahrzeugdaten" class="Str"("Value"=w223) -> ()  [unwired: 2 in, 2 out]
              }
            }
          }
        }
      }
      event "AFR, EGT": Value Change {
        n153 = event-data() -> ("NewVal"=w224:bool)  [unwired: 1 in, 5 out]
        n154 = local read "Y-Koord. Graph-Reset-Button (782)"() -> (w232:i32)
        n155 = local read "Höhe Leistungs-Graph (646)"() -> (w233:u32)
        n156 = control-ref of="Resetskalierung Leistung"() -> (w230:refnum<vi>)
        n157 = control-ref of="Autoskalierung Leistung"() -> (w225:refnum<vi>)
        n158 = control-ref of="AFR,EGT-Graph"() -> (w229:refnum<vi>)
        n159 = control-ref of="Leistungs-Graph"() -> (w231:refnum<vi>)
        n160 = control-ref of="Lambda"() -> (w226:refnum<vi>)
        n161 = property on="Autoskalierung AFR" class="Bool. (strikt)"("Visible"=w224) -> ()  [unwired: 2 in, 2 out]
        n162 = property on="Resetskalierung AFR" class="Bool. (strikt)"("Visible"=w224) -> ()  [unwired: 2 in, 2 out]
        n163 = control-ref of="AFR"() -> (w228:refnum<vi>)
        n164 = control-ref of="[°C]"() -> (w227:refnum<vi>)
        n165 = call "Enable_AFR_EGT_Graph (SubVI).vi"("Leistungsgraph"=w231, "AFR EGT"=w224, "Y-Koord. Graph-Reset-Button (782)"=w232, "Lambda"=w226, "Reset Skalierung"=w230, "Höhe Leistungs-Graph"=w233, "AFR EGT Gaph"=w229, "Auto Skalierung"=w225, "AFR"=w228, "EGT [°C]"=w227, "Skalierungsfaktor Leistungsgraph"=0.6666666666666666) -> ()  [unwired: 5 in]
      }
      event "Lambda": Value Change {
        w240 = 14.7
        w241 = 0.06802721088435375
        w257 = 0
        n166 = event-data() -> ("NewVal"=w242:bool)  [unwired: 1 in, 5 out]
        n167 = case shown="False" w242 {
          tunnel: ["AFR" "l"] -> w267
          tunnel: ["Anwendung" "Symbol"] -> w266
          tunnel: [20.0 1.6] -> w265
          tunnel: [10.0 0.4] -> w269
          tunnel: [w270 w275] -> w268
          tunnel: [w270 w275] -> w236
          frame False {
            w270 = 1
          }
          frame True {
            w275 = 2
          }
        }
        n168 = property on="AFR,EGT-Graph" class="XYGraph (strikt)"("ActYScl"=w257, "YScale.NameLbl.Text"=w267, "YScale.NameLbl.FontName"=w266, "YScale.Maximum"=w265, "YScale.Minimum"=w269, "YScale.Precision"=w268) -> ("Height"=w264:u32, "YScale.NameLbl.Width"=w263:u32, "Top"=w259:i32)  [unwired: 2 in, 2 out]
        n169 = property on="AFR" class="DigWert (strikt)"("Caption.Text"=w267, "Caption.FontName"=w266, "Format"=0, "Precision"=w236) -> ()  [unwired: 2 in, 2 out]
        n170 = Subtract(x=w264, y=w263) -> (x-y=w262:u32)
        n171 = local read "AFR,EGT-Graph"() -> (w253:cluster{dbl[], dbl[]}[])
        n172 = Divide(x=w262, y=2) -> (x/y=w260:dbl)
        n173 = Add(x=w260, y=w259) -> (x+y=w258:dbl)
        n174 = property on="AFR,EGT-Graph" class="XYGraph (strikt)"("ActYScl"=w257, "YScale.NameLbl.Top"=w258, "Active Plot"=0) -> ()  [unwired: 2 in, 2 out]
        n175 = Index Array(array=w253, index=1) -> (element=w245:cluster{dbl[], dbl[]})
        n176 = Index Array(array=w253, index=0) -> (element=w254:cluster{dbl[], dbl[]})
        n177 = local read "AFR"() -> (w239:dbl)
        n178 = Unbundle(w254) -> (w247:dbl[], w250:dbl[])
        n179 = Multiply(x=w241, y=w239) -> (x*y=w238:dbl)
        n180 = Multiply(x=w239, y=w240) -> (x*y=w237:dbl)
        n181 = Multiply(x=w241, y=w250) -> (x*y=w251:dbl[])
        n182 = Multiply(x=w240, y=w250) -> (x*y=w249:dbl[])
        n183 = Select(t=w251, s=w242, f=w249) -> (s? t:f=w248:dbl[])
        n184 = Select(t=w238, s=w242, f=w237) -> (s? t:f=w243:dbl)
        n185 = Bundle(w247, w248) -> (w246:cluster{dbl[], dbl[]})  [unwired: 1 in]
        n186 = local write "AFR"(w243) -> ()
        n187 = Build Array(w246, w245) -> (w244:cluster{dbl[], dbl[]}[])
        n188 = property on="AFR,EGT-Graph" class="XYGraph (strikt)"("Value"=w244) -> ()  [unwired: 2 in, 2 out]
      }
      event "Leistung": Value Change {
        w280 = 0.0
        n189 = event-data() -> ("NewVal"=w283:bool)  [unwired: 1 in, 5 out]
        n190 = case shown="True" w283 {
          tunnel: [w285 w288] -> w284
          tunnel: [w285 w289] -> w282
          frame False {
            w285 = T4."Disabled and Grayed Out" ("Deaktiviert")
          }
          frame True {
            w288 = T4."Enabled" ("Deaktiviert")
            n191 = local read "AFR, EGT"() -> (w287:bool)
            n192 = Select(t=w288, s=w287, f=T4."Disabled and Grayed Out" ("Deaktiviert")) -> (s? t:f=w289:T4)
          }
        }
        n193 = property on="Rear Tire\n[km/h]" class="Drehknopf (strikt)"("Value"=w280) -> ()  [unwired: 2 in, 2 out]
        n194 = property on="AFR" class="DigWert (strikt)"("Value"=w280) -> ()  [unwired: 2 in, 2 out]
        n195 = Bundle(w280, w280) -> (w281:cluster{dbl, dbl})  [unwired: 1 in]
        n196 = property on="[°C]" class="DigWert (strikt)"("Value"=w280) -> ()  [unwired: 2 in, 2 out]
        n197 = property on="Engine\n[1/min]" class="Drehknopf (strikt)"("Value"=w281) -> ()  [unwired: 2 in, 2 out]
        n198 = property on="AFR, EGT" class="Bool. (strikt)"("DisabledEnum"=w284) -> ()  [unwired: 2 in, 2 out]
        n199 = property on="Lambda" class="Bool. (strikt)"("DisabledEnum"=w282) -> ()  [unwired: 2 in, 2 out]
      }
      event "Resetskalierung AFR": Value Change {
        w295 = 0.0
        n200 = event-data() -> ()  [unwired: 1 in, 6 out]
        n201 = local read "Übersetzung ermitteln aus"() -> (w297:T2)
        n202 = local read "Lambda"() -> (w290:bool)
        n203 = case shown="Standard" w297 {
          tunnel: [14000.0 200.0] -> w296
          frame Default {
          }
          frame "vario (km/h)" {
          }
        }
        n204 = case shown="False" w290 {
          tunnel: [20.0 1.6] -> w292
          tunnel: [10.0 0.4] -> w291
          frame False {
          }
          frame True {
          }
        }
        n205 = property on="Leistungs-Graph" class="XYGraph (strikt)"("XScale.Maximum"=w296, "XScale.Minimum"=w295) -> ()  [unwired: 2 in, 2 out]
        n206 = property on="AFR,EGT-Graph" class="XYGraph (strikt)"("XScale.Maximum"=w296, "XScale.Minimum"=w295, "ActYScl"=w295, "YScale.Maximum"=w292, "YScale.Minimum"=w291, "ActYScl"=1, "YScale.Maximum"=800.0, "YScale.Minimum"=w295) -> ()  [unwired: 2 in, 2 out]
      }
      event "Autoskalierung Leistung": Value Change {
        w306 = 1  # Einmalige Autoskalierung
        n207 = event-data() -> ()  [unwired: 1 in, 6 out]
        n208 = property on="Leistungs-Graph" class="XYGraph (strikt)"("ActYScl"=0, "YScale.ScaleFit"=w306, "ActYScl"=1, "YScale.ScaleFit"=w306, "XScale.ScaleFit"=w306) -> ("XScale.Maximum"=w305:dbl, "XScale.Minimum"=w304:dbl)  [unwired: 2 in, 2 out]
        n209 = property on="AFR,EGT-Graph" class="XYGraph (strikt)"("XScale.Maximum"=w305, "XScale.Minimum"=w304) -> ()  [unwired: 2 in, 2 out]
      }
      event "Autoskalierung AFR": Value Change {
        w311 = 1  # Einmalige Autoskalierung
        n210 = event-data() -> ()  [unwired: 1 in, 6 out]
        n211 = property on="AFR,EGT-Graph" class="XYGraph (strikt)"("ActYScl"=0, "YScale.ScaleFit"=w311, "ActYScl"=1, "YScale.ScaleFit"=w311, "XScale.ScaleFit"=w311) -> ("XScale.Maximum"=w310:dbl, "XScale.Minimum"=w309:dbl)  [unwired: 2 in, 2 out]
        n212 = property on="Leistungs-Graph" class="XYGraph (strikt)"("XScale.Maximum"=w310, "XScale.Minimum"=w309) -> ()  [unwired: 2 in, 2 out]
      }
    }
    n213 = property class="Anw"() -> ("App.Kind"=w7:T6)  [unwired: 2 in, 2 out]
    n214 = Greater?(x=w7, y=1) -> (0:w8:bool)
    n215 = case shown="True" w8 {
      tunnel: w9 -> [_ w10]
      frame False {
      }
      frame True {
        n216 = Quit LabVIEW(quit? (T)=w10) -> ()
      }
    }
  }
  n217 = while {
    stop <- w319 stop-if-true
    n218 = Wait (ms)(milliseconds to wait=10) -> ()  [unwired: 1 out]
    n219 = local read "Übersetzung ermitteln aus"() -> (w317:T2)
    n220 = local read "Leistung"() -> (w318:bool)
    n221 = case shown="Standard" w317 {
      tunnel: [FALSE TRUE] -> w316
      frame Default {
      }
      frame "vario (km/h)" {
      }
    }
    n222 = case shown="False" w318 {
      tunnel: w316 -> [w331 _]
      frame False {
        n223 = control-ref of="Engine\n[1/min]"() -> (w335:refnum<vi>)
        n224 = control-ref of="Rear Tire\n[km/h]"() -> (w334:refnum<vi>)
        n225 = control-ref of="Ende"() -> (w333:refnum<vi>)
        n226 = control-ref of="Leistung"() -> (w332:refnum<vi>)
        n227 = control-ref of="[°C]"() -> (w327:refnum<vi>)
        n228 = control-ref of="AFR"() -> (w328:refnum<vi>)
        n229 = control-ref of="AFR, EGT"() -> (w330:refnum<vi>)
        n230 = control-ref of="Lambda"() -> (w329:refnum<vi>)
        n231 = call "Tachomodus (SubVI).vi"("Lambda"=w329, "Temp"=w327, "AFR EGT"=w330, "AFR"=w328, "cvt"=w331, "Leistung"=w332, "Stopp"=w333, "Hinterrad"=w334, "Welle"=w335) -> ()  [unwired: 3 in]
      }
      frame True {
      }
    }
    n232 = case shown="True" "record dyno speed" {
      frame False {
      }
      frame True {
        n233 = control-ref of="record dyno speed"() -> (w323:refnum<vi>)
        n234 = control-ref of="Ende"() -> (w322:refnum<vi>)
        n235 = control-ref of="Cyclecounter"() -> (w321:refnum<vi>)
        n236 = control-ref of="dT"() -> (w320:refnum<vi>)
        n237 = control-ref of="n(Rolle) [1/min]"() -> (w324:refnum<vi>)
        n238 = call "Rollendrehzahl (SubVI).vi"("dT(Rolle) (Eingang)"=w320, "Cyclecounter"=w321, "Stop"=w322, "Rollendrehzahl aufzeichnen"=w323, "n(Rolle) (Eingang)"=w324) -> ()  [unwired: 7 in]
      }
    }
    n239 = local read "Ende"() -> (w319:bool)
  }
  n240 = while {
    stop <- w343 stop-if-true
    n241 = local read "record dyno speed"() -> (w340:bool)
    n242 = Wait (ms)(milliseconds to wait=10) -> ()  [unwired: 1 out]
    n243 = Not(x=w340) -> (.not. x?=w339:bool)
    n244 = And(x="Leistung", y=w339) -> (x .and. y?=w337:bool)
    n245 = local read "Start"() -> (w344:bool)
    n246 = Not(x=w337) -> (.not. x?=w341:bool)
    n247 = case shown="True" w344 {
      tunnel: w337 -> [_ w387]
      frame False {
        w345 = T4."Enabled" ("Deaktiviert")
        n248 = property on="Leistung" class="Bool. (strikt)"("DisabledEnum"=w345) -> ()  [unwired: 2 in, 2 out]
        n249 = property on="record dyno speed" class="Bool. (strikt)"("DisabledEnum"=w345) -> ()  [unwired: 2 in, 2 out]
      }
      frame True {
        w368 = 0
        w369 = 0.0
        w371 = 0
        w374 = FALSE
        n250 = flat-sequence {
          tunnel: [w434] -> w419
          tunnel: [w433] -> w418
          tunnel: [w431] -> w417
          tunnel: w387 -> [w429]
          tunnel: [w427] -> w358
          tunnel: [w426] -> w357
          tunnel: [w427] -> w349
          tunnel: [w426] -> w348
          tunnel: w419 -> [w471]
          tunnel: w418 -> [w473]
          tunnel: [w467] -> w416
          tunnel: [w471] -> w415
          tunnel: [w473] -> w414
          tunnel: w417 -> [w472]
          tunnel: [w472] -> w413
          tunnel: [w463] -> w359
          tunnel: w358 -> [w463]
          tunnel: w357 -> [w462]
          tunnel: [w462] -> w356
          tunnel: [w489] -> w412
          tunnel: [w488] -> w386
          tunnel: [w487] -> w385
          tunnel: w416 -> [w489]
          tunnel: w415 -> [w485]
          tunnel: w414 -> [w484]
          tunnel: w413 -> [w486]
          tunnel: w359 -> [w481]
          tunnel: w356 -> [w480]
          tunnel: [w481] -> w355
          tunnel: [w480] -> w354
          tunnel: w412 -> [w501]
          tunnel: [w501] -> w411
          tunnel: [w500] -> w410
          tunnel: [w499] -> w409
          tunnel: [w497] -> w408
          tunnel: w386 -> [w500]
          tunnel: w385 -> [w499]
          tunnel: w355 -> [w493]
          tunnel: w354 -> [w494]
          tunnel: [w494] -> w353
          tunnel: [w493] -> w352
          tunnel: [w492] -> w347
          tunnel: [w491] -> w346
          tunnel: ["moving average Mittelwert"] -> w396
          tunnel: [w519] -> w397
          tunnel: [w518] -> w398
          tunnel: [w536] -> w399
          tunnel: [w530] -> w394
          tunnel: [w529] -> w395
          tunnel: [w537] -> w400
          tunnel: w411 -> [w537]
          tunnel: w410 -> [w532]
          tunnel: w409 -> [w531]
          tunnel: w408 -> [w536]
          tunnel: [w524] -> w384
          tunnel: [w525] -> w383
          tunnel: [w516] -> w380
          tunnel: w353 -> [w508]
          tunnel: w352 -> [w509]
          tunnel: [w509] -> w351
          tunnel: [w508] -> w350
          tunnel: w347 -> [w507]
          tunnel: w346 -> [w506]
          frame #0 {
            w439 = u16 0 items=["None", "XON/XOFF", "RTS/CTS", "XON/XOFF & RTS/CTS", "DTR/DSR", "XON/XOFF & DTR/DSR"] ("flow control (0:none)")
            w440 = u16 10 items=["1.0"=10, "1.5"=15, "2.0"=20] ("stop bits (10: 1 bit)")
            w432 = FALSE  # Enable Termination Char (T)
            w435 = u32 10000  # timeout (10sec)
            n251 = case shown="True" "Logfiles" {
              tunnel: [w444 w446] -> w427
              tunnel: [w444 w445] -> w426
              frame False {
                w444 = refnum<k0> refnum
              }
              frame True {
                w450 = 0  # read/write
                w451 = 4  # replace or create
                n252 = Open/Create/Replace File "Datei COM"(prompt="COM Logging", operation (0:open)=w451, access (0:read/write)=w450) -> (refnum out=w447:refnum<file>, error out=w448:errorcluster)  [unwired: 3 in, 1 out]
                n253 = case shown="Kein Fehler" w448 {
                  tunnel: w451 -> [w458 _]
                  tunnel: w450 -> [w457 _]
                  tunnel: w447 -> [w453 _]
                  tunnel: [w453 w461] -> w446
                  tunnel: [w452 w461] -> w445
                  frame No Error {
                    n254 = Open/Create/Replace File "Datei LV"(prompt="LabView Logging", operation (0:open)=w458, access (0:read/write)=w457) -> (refnum out=w455:refnum<file>, error out=w454:errorcluster)  [unwired: 3 in, 1 out]
                    n255 = case shown="Kein Fehler" w454 {
                      tunnel: [w459 refnum<k0> refnum] -> w452
                      tunnel: w455 -> [w459 _]
                      frame No Error {
                      }
                      frame Error {
                      }
                    }
                  }
                  frame Error {
                    w461 = refnum<k0> refnum
                  }
                }
              }
            }
            n256 = And(x="Messung Klimadaten", y=w429) -> (x .and. y?=w431:bool)
            n257 = call-poly "VISA Configure Serial Port"("VISA resource name"="Serielle Schnittstelle", "timeout (10sec)"=w435, "Enable Termination\nChar (T)"=w432, "baud rate (9600)"=u32 115200 ("baudrate (250000)"), "data bits (8)"=u16 8, "parity (0:none)"=enum16{"None", "Odd", "Even", "Mark", "Space"}."None", "stop bits (10: 1 bit)"=w440, "flow control (0:none)"=w439) -> ("VISA resource name out"=w437:refnum<visa-resource-name>, "error out"=w436:errorcluster)  [unwired: 6 in]
            n258 = VISA Clear(VISA resource name=w437, error in (no error)=w436) -> (VISA resource name out=w434:refnum<visa-resource-name>, error out=w433:errorcluster)
          }
          frame #1 {
            w466 = FALSE
            w464 = T4."Disabled and Grayed Out" ("Deaktiviert")
            w474 = 0.0  # Graphen löschen
            w467 = ""
            n259 = case shown="True" w472 {
              frame False {
                n260 = property on="Untersetzung\nermittelt" class="Bool. (strikt)"("Blinking"=TRUE ("Blinkend"), "BoolText.Text"="Initialisiere" ("Beschriftung.Text")) -> ()  [unwired: 2 in, 2 out]
              }
              frame True {
                n261 = Wait (ms)(milliseconds to wait=u32 2000 ("Zu wartende ms")) -> ()  [unwired: 1 out]
                n262 = property on="Untersetzung\nermittelt" class="Bool. (strikt)"("Blinking"=TRUE ("Blinkend"), "BoolText.Text"="Lese Klimadaten" ("Beschriftung.Text")) -> ()  [unwired: 2 in, 2 out]
              }
            }
            n263 = Build Array(w474) -> (w468:dbl[])
            n264 = property on="Auto-Gespeichert" class="Bool. (strikt)"("Value"=w466) -> ()  [unwired: 2 in, 2 out]
            n265 = property on="Lauf abgebrochen" class="Bool. (strikt)"("Value"=w466) -> ()  [unwired: 2 in, 2 out]
            n266 = property on="Untersetzung-Graph" class="SVDiagr (strikt)"("History Data"=w468) -> ()  [unwired: 2 in, 2 out]
            n267 = property on="Drucken" class="Bool. (strikt)"("DisabledEnum"=w464) -> ()  [unwired: 2 in, 2 out]
            n268 = property on="Übersetzung ermitteln aus" class="Enum (strikt)"("DisabledEnum"=w464) -> ()  [unwired: 2 in, 2 out]
            n269 = property on="Konfiguration:" class="Bool. (strikt)"("DisabledEnum"=w464) -> ()  [unwired: 2 in, 2 out]
            n270 = property on="Ende" class="Bool. (strikt)"("DisabledEnum"=w464) -> ()  [unwired: 2 in, 2 out]
            n271 = local write "Pmax"(w467) -> ()
            n272 = local write "COM-Fehlerrate"(w467) -> ()
            n273 = local write "Ergebnis"(w467) -> ()
            n274 = Bundle(w468, w468) -> (w470:cluster{dbl[], dbl[]})  [unwired: 1 in]
            n275 = Bundle(w468, w468) -> (w469:cluster{dbl[], dbl[]})  [unwired: 1 in]
            n276 = Build Array(w470, w469) -> (→"AFR,EGT-Graph" →"Leistungs-Graph":cluster{dbl[], dbl[]}[])
            n277 = local write "Auto-Datei"(w467) -> ()
            n278 = property on="Leistung" class="Bool. (strikt)"("DisabledEnum"=w464) -> ()  [unwired: 2 in, 2 out]
            n279 = property on="Speichern" class="Bool. (strikt)"("DisabledEnum"=w464) -> ()  [unwired: 2 in, 2 out]
            n280 = property on="record dyno speed" class="Bool. (strikt)"("DisabledEnum"=w464) -> ()  [unwired: 2 in, 2 out]
            n281 = property on="Logfiles" class="Bool. (strikt)"("DisabledEnum"=w464) -> ()  [unwired: 2 in, 2 out]
          }
          frame #2 {
            n282 = control-ref of="air temperature [°C]"() -> (w482:refnum<vi>)
            n283 = control-ref of="air pressure [mbar]"() -> (w483:refnum<vi>)
            n284 = call "MessungKlimadaten (SubVI).vi"("Datei LV (Eingang)"=w480, "Datei COM (Eingang)"=w481, "Boolesch"=w486, "Fehler (Eingang, kein Fehler)"=w484, "VISA resource name out"=w485, "Lufttemperatur [°C] (Eingang)"=w482, "Luftdruck [mbar] (Eingang)"=w483) -> ("Fehler (Ausgang)"=w487:errorcluster, "VISA-Referenz (Ausgang)"=w488:refnum<visa-resource-name>)  [unwired: 3 in]
          }
          frame #3 {
            n285 = local read "Lambda"() -> (w490:bool)
            n286 = Wait (ms)(milliseconds to wait=u32 2000 ("Zu wartende ms")) -> ()  [unwired: 1 out]
            n287 = case shown="True" w490 {
              tunnel: [20.0 1.6] -> w492
              tunnel: [10.0 0.4] -> w491
              frame False {
              }
              frame True {
              }
            }
            n288 = call "KorrekturfaktorDIN70020 (SubVI).vi"("Lufttemperatur [°C]"="air temperature [°C]", "Luftdruck [mbar]"="air pressure [mbar]") -> ("Korrekturfaktor"=w497:dbl)  [unwired: 9 in]
          }
          frame #4 {
            w514 = 1
            w513 = 0  # Keine Autoskalierung
            w510 = TRUE ("Kontinuierliche Aktualisierung")
            n289 = Concatenate Strings("m" ("String"), "\n") -> (w535:string)
            n290 = VISA Write(VISA resource name=w532, write buffer=w535, error in (no error)=w531) -> (VISA resource name out=w529:refnum<visa-resource-name>, error out=w530:errorcluster)  [unwired: 1 out]
            n291 = property on="Leistungs-Graph" class="XYGraph (strikt)"("ActYScl"=w513, "YScale.ScaleFit"=w513, "ActYScl"=w514, "YScale.ScaleFit"=w513, "XScale.ScaleFit"=w513, "Smooth Update"=w510) -> ()  [unwired: 2 in, 2 out]
            n292 = property on="AFR,EGT-Graph" class="XYGraph (strikt)"("ActYScl"=w513, "YScale.ScaleFit"=w513, "YScale.Maximum"=w507, "YScale.Minimum"=w506, "ActYScl"=w514, "YScale.ScaleFit"=w513, "YScale.Maximum"=800.0, "YScale.Minimum"=0.0, "XScale.ScaleFit"=w513, "Smooth Update"=w510) -> ()  [unwired: 2 in, 2 out]
            n293 = Divide(x="moving average Mittelwert", y=2) -> (x/y=w523:dbl)
            n294 = Round Toward -Infinity(1:w523) -> (0:w516:dbl)
            n295 = local read "difference quotient"() -> (w515:u8)
            n296 = call <vilib>:"Smoothing Filter Coefficients.vi"("shape"=1, "half-width"=w516, "type"=0) -> ("forward coefficients"=w519:dbl[], "reverse coefficients"=w518:dbl[])  [unwired: 6 in, 1 out]
            n297 = property on="Untersetzung\nermittelt" class="Bool. (strikt)"("Blinking"=FALSE ("Blinkend")) -> ()  [unwired: 2 in, 2 out]
            n298 = call <vilib>:"Smoothing Filter Coefficients.vi"("shape"=0, "half-width"=w515, "type"=0) -> ("forward coefficients"=w525:dbl[], "reverse coefficients"=w524:dbl[])  [unwired: 6 in, 1 out]
          }
        }
        n299 = Initialize Array(0.0 ("y"), 0) -> (w362:dbl[])
        n300 = Initialize Array(w368, w368) -> (w367:i32[])
        n301 = while {
          tunnel: w395 -> [w798]
          tunnel: w394 -> [w797]
          shift-right: [w841] -> _
          shift-left: w400 -> [w804]
          shift-right: [w757] -> _
          shift-left: w369 -> [w840]
          shift-right: [w836] -> _
          shift-left: w369 -> [w839]
          shift-right: [w732] -> _
          shift-left: w369 -> [w838]
          shift-right: [w773] -> _
          shift-left: w371 -> [w837]
          shift-right: [w810] -> w404
          shift-left: w369 -> [w792]
          shift-right: [w789] -> w402
          shift-left: w369 -> [w754]
          shift-right: [w807] -> _
          shift-left: w362 -> [w833]
          shift-right: [w733] -> _
          shift-left: w374 -> [w788]
          shift-right: [w830] -> w403
          shift-left: w362 -> [w828]
          shift-right: [w829] -> _
          shift-left: w362 -> [w746]
          shift-right: [w784] -> w376
          shift-left: w362 -> [w827]
          shift-right: [w824] -> _
          shift-left: w362 -> [w825]
          shift-right: [w823] -> w388
          shift-left: w362 -> [w826]
          shift-right: [w783] -> w377
          shift-left: w362 -> [w748]
          shift-right: [w782] -> w378
          shift-left: w362 -> [w749]
          tunnel: [w822] -> w407
          shift-right: [w818] -> w406
          shift-left: w371 -> [w820]
          tunnel: [w821] -> w391
          tunnel: [w787] -> w405
          tunnel: ["circum. dyno [m]"] -> w366
          shift-right: [w817] -> _
          shift-left: w374 -> [w796]
          shift-right: [w811] -> _
          shift-left: -5 -> [w816]
          shift-right: [w812] -> _
          shift-left: w369 -> [w815]
          shift-right: [w813] -> _
          shift-left: w369 -> [w814]
          shift-right: [w795] -> w365
          shift-left: w362 -> [w809]
          shift-right: [w727] -> _
          shift-left: _ -> [w806]
          shift-right: [w808] -> w401
          shift-left: w367 -> [w805]
          tunnel: [w803] -> w392
          tunnel: w399 -> [w759]
          tunnel: w398 -> [w799]
          tunnel: w397 -> [w781]
          tunnel: w396 -> [w758]
          tunnel: w384 -> [w794]
          tunnel: w383 -> [w793]
          shift-right: [w775] -> w381
          shift-left: w362 -> [w777]
          shift-right: [w774] -> w375
          shift-left: w362 -> [w747]
          tunnel: w380 -> [w766]
          tunnel: [w759] -> w379
          shift-right: [w714] -> _
          shift-left: _ -> [w739]
          shift-right: [w717] -> _
          shift-left: _ -> [w736]
          shift-right: [w740] -> w361
          shift-left: w362 -> [w743]
          shift-right: [w741] -> w360
          shift-left: w362 -> [w742]
          tunnel: w351 -> [w737]
          tunnel: w350 -> [w738]
          i -> [w779]
          stop <- w822 stop-if-true
          w715 = 0.0
          w731 = 0.06802721088435375  # AFR --> Lambda
          w772 = 3  # Vario(km/h)
          n302 = property class="Instr"(reference=w798, error in=w797) -> (reference out=w802:refnum<visa-resource-name>, error out=w801:errorcluster, "Serial Settings:Number of Bytes at Serial Port"=w762:u32)
          n303 = Greater?(x=w762, y=u32 1 ("min. Bytes")) -> (0:w763:bool)
          n304 = Select(t=w762, s=w763, f=u32 0 ("Bytes at Port")) -> (s? t:f=w761:u32)
          n305 = control-ref of="Füllstand Lesepuffer"() -> (w786:refnum<vi>)
          n306 = property on="AFR, EGT" class="Bool. (strikt)"() -> ("Value"=w713:bool)  [unwired: 2 in, 2 out]
          n307 = call "Stringhandling (SubVI).vi"("Slide (Eingang)"=w786, "Füllstand Lesepuffer (Eingang)"=w837, "Datei COM (Eingang)"=w737, "VISA-Referenz (Eingang)"=w802, "MessFrequenz [Hz] (Eingang)"=w838, "Bytes at Port"=w761, "Datei LV (Eingang)"=w738, "Fehler (Eingang, kein Fehler)"=w801, "Cyclecounter (Eingang)"=w806, "Rolle[Hz] (Eingang)"=w839, "Temp[°C] (Eingang)"=w739, "AFR (Eingang)"=w736, "String (Eingang)"=w804, "Zündung [Hz] (Eingang)"=w840) -> ("Lesepuffer"=→"Lesepuffer":string, "Füllstand Lesepuffer (Ausgang)"=w773:i32, "String (Ausgang)"=w841:string, "Temp[°C] (Ausgang)"=w714:dbl, "AFR (Ausgang)"=w717:dbl, "VISA-Referenz (Ausgang)"=w803:refnum<visa-resource-name>, "Zündung [Hz] (Ausgang)"=w756:dbl, "Rolle [Hz] (Ausgang)"=w836:dbl, "Messfrequenz [Hz] (Ausgang)"=w732:dbl, "Cyclecounter (Ausgang)"=w727:i32, "Fehler (Ausgang)"=w821:errorcluster)  [unwired: 3 in]
          "Füllstand Lesepuffer" <- w773
          "Cyclecounter" <- w727
          n308 = Select(t=w717, s=w713, f=w715) -> (s? t:f=w718:dbl)
          n309 = local read "Übersetzung ermitteln aus"() -> (w771:T2)
          n310 = Multiply(x=0.06802721088435375, y=w718) -> (x*y=w720:dbl)
          n311 = local read "Lambda"() -> (w721:bool)
          n312 = Not Equal?(x=w772, y=w771) -> (x != y?=w769:bool)
          n313 = Select(t=w720, s=w721, f=w718) -> (s? t:f=→"AFR":dbl)
          n314 = And(x="Filter Zündsignal", y=w769) -> (x .and. y?=w767:bool)
          n315 = Select(t=w766, s=w767, f=0) -> (s? t:f=w755:dbl)
          n316 = call <vilib>:"Median Filter PtByPt.vi"("initialize"=TRUE, "rank"=w755, "x"=w756) -> ("Filtered x"=w757:dbl)  [unwired: 1 in, 1 out]
          n317 = Not Equal?(x=w806, y=w727) -> (x != y?=w724:bool)
          n318 = Select(t=w714, s=w713, f=w715) -> (s? t:f=→"[°C]":dbl)
          n319 = case shown="\"vario (km/h)\"" w771 {
            tunnel: [w876 "n min [1/min]"] -> w787
            frame "vario (km/h)" {
              n320 = local read "circum. dyno [m]"() -> (w877:dbl)
              n321 = Divide(x="v min [km/h]", y=w877) -> (x/y=w875:dbl)
              n322 = Multiply(x=w875, y=16.66666667) -> (x*y=w876:dbl)
            }
            frame Default {
            }
          }
          n323 = case "Case-Struktur" shown="True" w724 {
            tunnel: w757 -> [w1140 w1162]
            tunnel: w836 -> [w1139 w1161]
            tunnel: [w1140 w1152] -> w835
            tunnel: [w1139 w1149] -> w834
            tunnel: w732 -> [_ w1157]
            tunnel: w792 -> [w1138 _]
            tunnel: [w1138 w1148] -> w810
            tunnel: w754 -> [_ w1150]
            tunnel: "circum. dyno [m]" -> [_ w1160]
            tunnel: w771 -> [_ w1156]
            tunnel: [w1136 w1144] -> w730
            tunnel: [w1137 w1142] -> w729
            frame False {
              n324 = local read "Engine\n[1/min]"() -> (w1136:cluster{dbl, dbl})
              n325 = local read "Rear Tire\n[km/h]"() -> (w1137:dbl)
            }
            frame True {
              w1164 = 60.0 ("y")
              n326 = Reciprocal "Abtastzeit [s]"(x=w1157) -> (1/x=w1148:dbl)
              "dT" <- w1148
              n327 = Divide "R [1/s]"(x=w1161, y="incr./rev. dyno  [Inkr/U]") -> (x/y=w1151:dbl)
              n328 = Divide(x=w1162, y="ignition [Imp/rev]") -> (x/y=w1163:dbl)
              n329 = Multiply "[m/s]"(x=w1151, y=w1160) -> (x*y=w1141:dbl)
              n330 = Multiply(x=w1141, y=w1148) -> (x*y=w1145:dbl)
              n331 = Multiply "nZ gemessen [1/min]"(x=w1163, y=w1164) -> (x*y=w1152:dbl)
              n332 = Multiply "nR [1/min]"(x=w1164, y=w1151) -> (x*y=w1149:dbl)
              "n(Rolle) [1/min]" <- w1149
              n333 = local read "Strecke [m]"() -> (w1146:dbl)
              n334 = Multiply "nZ berechnet [1/min]"(x=w1150, y=w1149) -> (x*y=w1154:dbl)
              n335 = Add(x=w1146, y=w1145) -> (x+y=→"Strecke [m]":dbl)
              n336 = case shown="Standard" w1156 {
                tunnel: [w1166 w1167] -> w1155
                tunnel: w1154 -> [w1166 w1168]
                tunnel: [w1165 w1168] -> w1153
                tunnel: w1152 -> [w1165 w1167]
                frame Default {
                }
                frame "vario (km/h)" {
                }
              }
              n337 = Multiply ("[km/h]")(x=3.6 ("y"), y=w1141) -> (x*y=w1142:dbl)
              n338 = Bundle(w1155, w1153) -> (w1144:cluster{dbl, dbl})  [unwired: 1 in]
            }
          }
          n339 = case shown="True" w724 {
            tunnel: w816 -> [w887 w898]
            tunnel: [w887 w910] -> w811
            tunnel: w815 -> [w886 w909]
            tunnel: [w886 w895] -> w812
            tunnel: w814 -> [w885 w908]
            tunnel: [w885 w896] -> w813
            tunnel: w727 -> [_ w894]
            tunnel: w805 -> [w884 w893]
            tunnel: [w884 w897] -> w808
            frame False {
            }
            frame True {
              n340 = Build Array (concatenate)(w893, w894) -> (w897:i32[])
              n341 = Greater Or Equal To 0?(x=w898) -> (x >= 0?=w899:bool)
              n342 = case shown="True" w899 {
                tunnel: [w911 w922] -> w895
                tunnel: [w911 w923] -> w896
                tunnel: [w912 w914] -> w910
                tunnel: w909 -> [_ w916]
                tunnel: w908 -> [_ w924]
                tunnel: w894 -> [w912 w913]
                tunnel: w898 -> [_ w914]
                frame False {
                  w911 = 1.0
                }
                frame True {
                  w920 = 65536.0
                  n343 = Add(x=w914, y=w916) -> (x+y=w915:dbl)
                  n344 = Divide(x=w915, y=w920) -> (x/y=w925:dbl)
                  n345 = Increment(x=w924) -> (x+1=w923:dbl)
                  n346 = Round Toward -Infinity(1:w925) -> (0:w921:dbl)
                  n347 = Multiply(x=w921, y=w920) -> (x*y=w919:dbl)
                  n348 = Add(x=w919, y=w913) -> (x+y=w918:dbl)
                  n349 = Increment(x=w918) -> (x+1=w917:dbl)
                  n350 = Subtract(x=w917, y=w914) -> (x-y=w922:dbl)
                }
              }
              n351 = Subtract(x=w895, y=w896) -> (x-y=w890:dbl)
              n352 = Decrement(x=w890) -> (x-1=w889:dbl)
              n353 = Max & Min(x=0, y=w889) -> (max(x,y)=w888:dbl)  [unwired: 1 out]
              n354 = Divide(x=w888, y=w895) -> (x/y=w902:dbl)
              n355 = Greater Than 0?(x=w888) -> (x > 0?=w892:bool)
              n356 = Select(t=u32 16711680, s=w892, f=u32 0) -> (s? t:f=w903:u32)
              n357 = Multiply(x=w902, y=100.0) -> (x*y=w900:dbl)
              n358 = property on="COM-Fehlerrate" class="Str"("Text.TextColor"=w903) -> ()  [unwired: 2 in, 2 out]
              n359 = Format Into String(format string="%d / %.1f%%" ("Format-String"), w888, w900) -> (resulting string=→"COM-Fehlerrate":string)  [unwired: 2 in, 1 out]
            }
          }
          n360 = Quotient & Remainder(x=w727, y=2) -> (x-y*floor(x/y)=w726:i32)  [unwired: 1 out]
          n361 = Equal To 0?(x=w726) -> (x = 0?=w725:bool)
          n362 = And(x=w724, y=w725) -> (x .and. y?=w723:bool)
          n363 = case shown="True" w723 {
            tunnel: w730 -> [_ w843]
            tunnel: w729 -> [_ w842]
            frame False {
            }
            frame True {
              "Engine\n[1/min]" <- w843
              "Rear Tire\n[km/h]" <- w842
            }
          }
          n364 = case shown="True" w724 {
            tunnel: w835 -> [_ w986]
            tunnel: w834 -> [_ w1039]
            tunnel: "circum. dyno [m]" -> [_ w1040]
            tunnel: [w941 w969] -> w789
            tunnel: w754 -> [w930 w969]
            tunnel: w788 -> [w942 w988]
            tunnel: w833 -> [w943 w1043]
            tunnel: [w942 w1015] -> w733
            tunnel: [w943 w1042] -> w807
            tunnel: w799 -> [_ w985]
            tunnel: w781 -> [_ w984]
            tunnel: [w940 w966] -> w830
            tunnel: [w939 w967] -> w829
            tunnel: w828 -> [w940 w1038]
            tunnel: w746 -> [w939 _]
            tunnel: w758 -> [_ w983]
            tunnel: [w938 w973] -> w784
            tunnel: w827 -> [w938 _]
            tunnel: [w937 w996] -> w824
            tunnel: w825 -> [w937 _]
            tunnel: [w936 w980] -> w823
            tunnel: w826 -> [w936 _]
            tunnel: [w935 w974] -> w783
            tunnel: w748 -> [w935 _]
            tunnel: [w934 w1032] -> w782
            tunnel: w749 -> [w934 _]
            tunnel: w759 -> [_ w982]
            tunnel: w820 -> [w933 w1026]
            tunnel: w787 -> [_ w1017]
            tunnel: [w933 w1025] -> w818
            tunnel: w796 -> [w932 w1022]
            tunnel: [w932 w1021] -> w817
            tunnel: w810 -> [_ w1020]
            tunnel: [w931 w990] -> w795
            tunnel: w809 -> [w931 w1019]
            tunnel: w794 -> [_ w1003]
            tunnel: w793 -> [_ w1002]
            tunnel: w777 -> [w929 w987]
            tunnel: [w929 w968] -> w775
            tunnel: [w928 w964] -> w774
            tunnel: w747 -> [w928 _]
            tunnel: w766 -> [_ w965]
            tunnel: [w927 w963] -> w740
            tunnel: w743 -> [w927 w962]
            tunnel: w717 -> [_ w961]
            tunnel: [w926 w960] -> w741
            tunnel: w714 -> [_ w959]
            tunnel: w742 -> [w926 w958]
            frame False {
              n365 = case shown="False" w942 {
                tunnel: w943 -> [w950 _]
                tunnel: [w944 w957] -> w941
                tunnel: w930 -> [_ w957]
                frame False {
                  n366 = local read "Übersetzung ermitteln aus"() -> (w947:T2)
                  n367 = call <vilib>:"Measures of Mean.vi"("percent (trim)"=20.0, "type"=3, "x array"=w950) -> ("mean value"=w945:dbl)  [unwired: 7 in, 1 out]
                  n368 = Equal To 0? "aus Zündsignal?"(x=w947) -> (x = 0?=w946:bool)
                  n369 = case shown="True" w946 {
                    tunnel: w945 -> [w951 w956]
                    tunnel: [w951 w952] -> w944
                    frame False {
                    }
                    frame True {
                      w953 = 1000.0
                      n370 = Multiply(x=w956, y=w953) -> (x*y=w955:dbl)
                      n371 = Round To Nearest(number=w955) -> (nearest integer value=w954:dbl)
                      n372 = Divide(x=w954, y=w953) -> (x/y=w952:dbl)
                    }
                  }
                }
                frame True {
                }
              }
            }
            frame True {
              w1029 = 0.00135962  # [W] in [PS]
              w1034 = 0.10471975511965978  # 2*Pi/60
              # "Einzelne Ausreisser (Zündsignal) werden\nam besten mit Median-Filter eliminiert"
              n373 = Not(x=w988) -> (.not. x?=w993:bool)
              n374 = local read "Leistung"() -> (w992:bool)
              n375 = Or(x=w992, y=w993) -> (x .or. y?=w991:bool)
              n376 = Square(x=w969) -> (x^2=w1033:dbl)
              n377 = local read "Übersetzung ermitteln aus"() -> (w994:T2)
              n378 = case shown="True" w991 {
                tunnel: w1039 -> [_ w1063]
                tunnel: w1038 -> [w1047 w1062]
                tunnel: w1020 -> [_ w1061]
                tunnel: w1019 -> [w1048 w1060]
                tunnel: [w1047 w1059] -> w966
                tunnel: [w1048 w1058] -> w990
                tunnel: w987 -> [w1046 w1057]
                tunnel: [w1046 w1056] -> w968
                tunnel: w986 -> [_ w1055]
                tunnel: [w1045 w1054] -> w963
                tunnel: w962 -> [w1045 w1053]
                tunnel: w961 -> [_ w1052]
                tunnel: [w1044 w1051] -> w960
                tunnel: w959 -> [_ w1049]
                tunnel: w958 -> [w1044 w1050]
                frame False {
                }
                frame True {
                  n379 = Build Array (concatenate) "nRolle in Array einf."(w1062, w1063) -> (w1059:dbl[])
                  n380 = Build Array (concatenate) "nWelle in Array einf."(w1057, w1055) -> (w1056:dbl[])
                  n381 = Build Array (concatenate) "dT in Array einf."(w1060, w1061) -> (w1058:dbl[])
                  n382 = Build Array (concatenate) "AFR in Array einf."(w1053, w1052) -> (w1054:dbl[])
                  n383 = Build Array (concatenate) "EGT in Array einf."(w1050, w1049) -> (w1051:dbl[])
                }
              }
              n384 = Divide(x="Inertia dyno [kgm²]", y=w1033) -> (x/y=w981:dbl)
              n385 = case shown="\"ignition signal\"" w994 {
                tunnel: w986 -> [w1128 _ _ _]
                tunnel: w1039 -> [w1127 _ _ _]
                tunnel: [w1126 w1132 "nCrank/nDyno" 1.0] -> w1041
                tunnel: w1040 -> [_ w1133 _ _]
                frame "ignition signal" {
                  n386 = Divide(x=w1128, y=w1127) -> (x/y=w1126:dbl)
                }
                frame "gear ratio & speed" {
                  n387 = Divide(x=w1133, y="tire circumferential  [m]") -> (x/y=w1131:dbl)
                  n388 = Multiply(x=w1131, y="gear ratio [1:]") -> (x*y=w1132:dbl)
                }
                frame "nCrank / nDyno" {
                }
                frame "vario (km/h)" {
                }
              }
              n389 = Multiply(x=w982, y=w981) -> (x*y=w979:dbl)
              n390 = local read "difference quotient"() -> (w1001:u8)
              n391 = Index Array(array=w966, index=1 ("Index")) -> (element=w1013:dbl)
              n392 = Index Array(array=w990, index=1 ("Index")) -> (element=w1007:dbl)
              n393 = Multiply(x=2, y=w1001) -> (x*y=w999:i32)
              n394 = Initialize Array(w1013, w983) -> (w1012:dbl[])
              n395 = Increment(x=w999) -> (x+1=w997:i32)
              n396 = Initialize Array(w1007, w997) -> (w1005:dbl[])
              n397 = Insert Into Array(array=w966, index=0 ("Index"), new element=w1012) -> (w1010:dbl[])
              n398 = Insert Into Array(array=w990, index=0 ("Index"), new element=w1005) -> (w1004:dbl[])
              n399 = call-poly <vilib>:"IIR Filter.vi"("Forward Coefficients"=w984, "Reverse Coefficients"=w985, "X"=w1010) -> ("Filtered X"=w1009:dbl[])  [unwired: 1 in, 1 out]
              n400 = call-poly <vilib>:"IIR Filter.vi"("Forward Coefficients"=w1002, "Reverse Coefficients"=w1003, "X"=w1004) -> ("Filtered X"=w998:dbl[])  [unwired: 1 in, 1 out]
              n401 = case shown="False" w988 {
                selector: w988 -> [_ w1125]
                tunnel: w1041 -> [w1113 _]
                tunnel: w1043 -> [w1115 w1124]
                tunnel: [w1110 w1125] -> w1037
                tunnel: [w1114 w1124] -> w1042
                tunnel: w1022 -> [w1112 w1123]
                tunnel: [w1110 w1123] -> w1021
                tunnel: w994 -> [w1109 _]
                frame False {
                  n402 = Build Array (concatenate)(w1115, w1113) -> (w1114:dbl[])
                  n403 = case shown="\"ignition signal\"" w1109 {
                    tunnel: ["duration  [s]" 0.0 ("Dauer [s]")] -> w1111
                    frame "ignition signal" {
                      n404 = property on="Untersetzung\nermittelt" class="Bool. (strikt)"("Blinking"=TRUE ("Blinkend"), "BoolText.Text"="Ermittle Übersetzung" ("Boolescher Text.Text")) -> ()  [unwired: 2 in, 2 out]
                    }
                    frame Default {
                    }
                  }
                  n405 = call "Verstrichene Zeit"("Time Target (s)"=w1111, "Reset"=w1112) -> ("Time has Elapsed"=w1110:bool)  [unwired: 10 in, 7 out]
                  n406 = case shown="True" w1110 {
                    frame False {
                    }
                    frame True {
                      n407 = property on="Untersetzung\nermittelt" class="Bool. (strikt)"("Blinking"=FALSE ("Blinkend"), "BoolText.Text"="Go" ("Boolescher Text.Text")) -> ()  [unwired: 2 in, 2 out]
                      n408 = property on="Strecke [m]" class="DigWert (strikt)"("Value"=0.0) -> ()  [unwired: 2 in, 2 out]
                    }
                  }
                  "Untersetzung-Graph" <- w1113
                }
                frame True {
                }
              }
              n409 = Array Subset "Rolle gefiltert [1/min]"(array=w1009, index=w983) -> (w967:dbl[])  [unwired: 1 in]
              n410 = Array Subset "dT gefiltert [s]"(array=w998, index=w997) -> (w995:dbl[])  [unwired: 1 in]
              n411 = Array Size "Array-Größe"(array=w967) -> (size(s)=w1035:i32)
              n412 = Greater?(x=w1035, y=w983) -> (0:w1036:bool)
              n413 = call <vilib>:"Median Filter.vi"("right rank"=w965, "left rank"=w965, "X"=w968) -> ("Filtered X"=w964:dbl[])  [unwired: 7 in, 1 out]
              n414 = Multiply "* i"(x=w967, y=w969) -> (x*y=w973:dbl[])
              n415 = Multiply(x=w973, y=w1034) -> (x*y=w996:dbl[])
              n416 = And(x=w1037, y=w1036) -> (x .and. y?=w1015:bool)
              n417 = Array Size "Array-Größe"(array=w996) -> (size(s)=w989:i32)
              n418 = Decrement(x=w989) -> (x-1=w1027:i32)
              n419 = Select(t=w1017, s=w1015, f=1000000.0) -> (s? t:f=w1018:dbl)
              n420 = Initialize Array(0.0 ("y"), 0) -> (w975:dbl[])
              n421 = for {
                N: w989 -> [_]
                tunnel: "difference quotient" -> [w1086]
                tunnel: w996 -> [w1093]
                tunnel: w1027 -> [w1085]
                shift-right: [w1090] -> w980
                shift-left: w975 -> [w1091]
                tunnel: w973 -> [w1068] mode=indexing
                tunnel: w1026 -> [w1078]
                tunnel: w1018 -> [w1088]
                tunnel: [w1079] -> w1025
                tunnel: w988 -> [w1077]
                tunnel: w995 -> [w1074] mode=indexing
                tunnel: "dynospeed of torque loss. n1 [1/min]" -> [w1071]
                tunnel: "torque loss M1 [Nm] @ n1" -> [w1070]
                tunnel: "torque loss M0 [Nm] @ n = 0" -> [w1069]
                shift-right: [w1067] -> w972
                shift-left: w975 -> [w1066]
                tunnel: w967 -> [w1064] mode=indexing
                i -> [w1075]
                stop <- w1072 stop-if-true
                # "Beschleunigung a(i) berechnen solange bis n(i) > nSchwelle & a(i) < 0"
                n422 = call "Verlustmoment (SubVI).vi"("n [1/min"=w1064, "Verlustmoment M0 [Nm] bei n = 0"=w1069, "Verlustmoment M1 [Nm] bei n1"=w1070, "Rollendrehzahl n1 [1/min]"=w1071) -> ("Mv"=w1065:dbl)  [unwired: 7 in]
                n423 = Subtract(x=w1085, y=w1086) -> (x-y=w1087:i32)
                n424 = Multiply(x=w1074, y=2.0) -> (x*y=w1076:dbl)
                n425 = Subtract(x=w1075, y=w1086) -> (x-y=w1106:i32)
                n426 = Add(x=w1075, y=w1086) -> (x+y=w1100:i32)
                n427 = Greater Or Equal?(x=w1075, y=w1086) -> (x >= y?=w1082:bool)
                n428 = Less Or Equal?(x=w1075, y=w1087) -> (x <= y?=w1083:bool)
                n429 = Greater?(x=w1068, y=w1088) -> (0:w1089:bool)
                n430 = Max & Min(x=w1085, y=w1100) -> (min(x,y)=w1101:i32)  [unwired: 1 out]
                n431 = Max & Min(x=w1106, y=0) -> (max(x,y)=w1104:i32)  [unwired: 1 out]
                n432 = Subtract(x=w1101, y=w1075) -> (x-y=w1102:i32)
                n433 = Subtract(x=w1075, y=w1104) -> (x-y=w1103:i32)
                n434 = Max & Min(x=w1103, y=w1102) -> (min(x,y)=w1094:i32)  [unwired: 1 out]
                n435 = Add(x=w1075, y=w1094) -> (x+y=w1099:i32)
                n436 = Subtract(x=w1075, y=w1094) -> (x-y=w1098:i32)
                n437 = Multiply(x=w1094, y=w1076) -> (x*y=w1092:dbl)
                n438 = Index Array(array=w1093, index=w1099) -> (element=w1096:dbl)
                n439 = Index Array(array=w1093, index=w1098) -> (element=w1097:dbl)
                n440 = Subtract(x=w1096, y=w1097) -> (x-y=w1095:dbl)
                n441 = Divide(x=w1095, y=w1092) -> (x/y=w1084:dbl)
                n442 = Less Than 0?(x=w1084) -> (x < 0?=w1081:bool)
                n443 = Less Or Equal To 0?(x=w1078) -> (x <= 0?=w1080:bool)
                n444 = Build Array (concatenate)(w1091, w1084) -> (w1090:dbl[])
                n445 = Compound Arithmetic op=AND "n(i) > nSchwelle\n& a(i) < 0"(w1081, w1089, w1080, w1082, w1083, w1077) -> (w1072:bool)
                n446 = case shown="False" w1072 {
                  tunnel: w1075 -> [_ w1108]
                  tunnel: [w1107 w1108] -> w1079
                  tunnel: w1078 -> [w1107 _]
                  frame False {
                  }
                  frame True {
                  }
                }
                n447 = Build Array (concatenate) "Mv Rolle"(w1066, w1065) -> (w1067:dbl[])
              }
              n448 = Divide ": i"(x=w972, y=w969) -> (x/y=w971:dbl[])
              n449 = Multiply "* J' * korr"(x=w979, y=w980) -> (x*y=w970:dbl[])
              n450 = Add(x=w970, y=w971) -> (x+y=w974:dbl[])
              n451 = Multiply(x=w996, y=w974) -> (x*y=w1028:dbl[])
              n452 = Multiply(x=w1029, y=w1028) -> (x*y=w1032:dbl[])
            }
          }
          "Untersetzung\nermittelt" <- w733
          n453 = local read "Übersetzung ermitteln aus"() -> (w776:T2)
          n454 = Quotient & Remainder(x=w779, y=500) -> (x-y*floor(x/y)=w780:i32)  [unwired: 1 out]
          n455 = Equal To 0? "aus Zündsignal?"(x=w776) -> (x = 0?=w791:bool)
          n456 = Equal To 0?(x=w780) -> (x = 0?=w734:bool)
          n457 = And(x=w733, y=w734) -> (x .and. y?=w735:bool)
          n458 = local read "Leistung"() -> (w751:bool)
          n459 = local read "record dyno speed"() -> (w753:bool)
          n460 = And(x=w733, y=w791) -> (x .and. y?=w790:bool)
          n461 = case shown="True" w735 {
            tunnel: w784 -> [_ w869]
            tunnel: w783 -> [_ w860]
            tunnel: w782 -> [_ w865]
            tunnel: w776 -> [_ w862]
            tunnel: "circum. dyno [m]" -> [_ w868]
            tunnel: w774 -> [_ w859]
            tunnel: w741 -> [_ w851]
            tunnel: w740 -> [_ w846]
            tunnel: w731 -> [_ w847]
            frame False {
            }
            frame True {
              # "Livegraph"
              # "Skal-Y2"
              # "Skal-Y1"
              # "Skal-X"
              n462 = call "n2v (SubVI).vi"("Übersetzung ermitteln aus"=w862, "Array (Eingang)"=w869, "Rollenumfang [m]"=w868) -> ("Array (Ausgang)"=w848:dbl[])  [unwired: 7 in, 1 out]
              n463 = control-ref of="Leistungs-Graph"() -> (w855:refnum<vi>)
              n464 = case shown="Standard" w862 {
                tunnel: [w871 w873] -> w861
                tunnel: w860 -> [w871 _]
                tunnel: w859 -> [_ w873]
                tunnel: [w871 w873] -> w858
                tunnel: [10.0 1000.0] -> w856
                frame Default {
                }
                frame "vario (km/h)" {
                }
              }
              n465 = call "ScaleGraphY (SubVI).vi"("AktYSkl"=1, "Divisor"=w856, "Array"=w858, "Faktor"=1.8, "XYGraph (Eingang)"=w855) -> ()  [unwired: 7 in]
              n466 = local read "Lambda"() -> (w850:bool)
              n467 = call "ScaleGraphY (SubVI).vi"("AktYSkl"=0, "Divisor"=10.0, "Array"=w865, "Faktor"=1.0, "XYGraph (Eingang)"=w855) -> ()  [unwired: 7 in]
              n468 = call "ScaleGraphX (SubVI).vi"("Array"=w848, "Übersetzung ermitteln aus"=w862, "XYGraph (Eingang)"=w855) -> ("xMax (Ausgang)"=w853:dbl, "xMin (Ausgang)"=w854:dbl)  [unwired: 7 in]
              n469 = control-ref of="AFR,EGT-Graph"() -> (w852:refnum<vi>)
              n470 = Multiply(x=w846, y=w847) -> (x*y=w845:dbl[])
              n471 = property on="AFR,EGT-Graph" class="XYGraph (strikt)"("XScale.Minimum"=w854, "XScale.Maximum"=w853) -> ()  [unwired: 2 in, 2 out]
              n472 = Select(t=w845, s=w850, f=w846) -> (s? t:f=w849:dbl[])
              n473 = call "UpdateGraph (SubVI).vi"("x"=w848, "Y2"=w861, "Y1"=w865, "XYGraph (Eingang)"=w855) -> ()  [unwired: 8 in]
              n474 = call "UpdateGraph (SubVI).vi"("x"=w848, "Y2"=w851, "Y1"=w849, "XYGraph (Eingang)"=w852) -> ()  [unwired: 8 in]
            }
          }
          n475 = Select(t=w789, s=w733, f=0.0) -> (s? t:f=→"Untersetzung":dbl)
          n476 = case shown="True" w790 {
            tunnel: w789 -> [_ w883]
            frame False {
            }
            frame True {
              n477 = local write "nCrank/nDyno"(w883) -> ()
            }
          }
          n478 = Not(x=w753) -> (.not. x?=w752:bool)
          n479 = And(x=w751, y=w752) -> (x .and. y?=w750:bool)
          n480 = case shown="True" w750 {
            tunnel: [FALSE w882] -> w819
            tunnel: w818 -> [_ w881]
            frame False {
            }
            frame True {
              n481 = Greater Than 0?(x=w881) -> (x > 0?=w882:bool)
            }
          }
          n482 = local read "Start"() -> (w800:bool)
          n483 = Not(x=w800) -> (.not. x?=w745:bool)
          n484 = case shown="True" w745 {
            frame False {
            }
            frame True {
              n485 = property on="Lauf abgebrochen" class="Bool. (strikt)"("Value"=TRUE) -> ()  [unwired: 2 in, 2 out]
            }
          }
          n486 = Or(x=w819, y=w745) -> (x .or. y?=w822:bool)
        }
        n487 = VISA Clear(VISA resource name=w392, error in (no error)=w391) -> (VISA resource name out=w389:refnum<visa-resource-name>, error out=w393:errorcluster)
        n488 = VISA Close(VISA resource name=w389, error in (no error)=w393) -> ()  [unwired: 1 out]
        n489 = case shown="True" w407 {
          tunnel: w376 -> [_ w627]
          tunnel: w377 -> [_ w628]
          tunnel: w378 -> [_ w629]
          tunnel: w406 -> [_ w617]
          tunnel: w388 -> [_ w665]
          tunnel: w405 -> [_ w664]
          tunnel: w366 -> [_ w644]
          tunnel: w379 -> [_ w638]
          tunnel: w402 -> [_ w650]
          tunnel: w375 -> [_ w626]
          tunnel: w361 -> [_ w619]
          tunnel: w360 -> [_ w618]
          frame False {
          }
          frame True {
            w645 = 0.06
            n490 = Array Subset "P"(array=w629, length=w617) -> (w633:dbl[])  [unwired: 1 in]
            n491 = Array Subset "M"(array=w628, length=w617) -> (w632:dbl[])  [unwired: 1 in]
            n492 = Array Subset "alpha"(array=w665, length=w617) -> (w666:dbl[])  [unwired: 1 in]
            n493 = Array Subset "nWelle"(array=w626, length=w617) -> (w630:dbl[])  [unwired: 1 in]
            n494 = Array Subset "AFR"(array=w619, length=w617) -> (w616:dbl[])  [unwired: 1 in]
            n495 = Array Subset "EGT"(array=w618, length=w617) -> (w615:dbl[])  [unwired: 1 in]
            n496 = Array Subset "n"(array=w627, length=w617) -> (w631:dbl[])  [unwired: 1 in]
            n497 = local read "Lambda"() -> (w606:bool)
            n498 = Array Size(array=w666) -> (size(s)=w667:i32)
            n499 = for {
              N: w667 -> [w712]
              tunnel: w665 -> [w709]
              tunnel: w627 -> [w706]
              tunnel: w664 -> [w703]
              tunnel: [w701] -> w656
              i -> [w707]
              stop <- w702 stop-if-true
              # "Beginn mit n(i)<nSchwelle &  a(i)<0 wegschneiden"
              n500 = Decrement(x=w712) -> (x-1=w711:i32)
              n501 = Subtract(x=w711, y=w707) -> (x-y=w701:i32)
              n502 = Index Array(array=w706, index=w701) -> (element=w705:dbl)
              n503 = Index Array(array=w709, index=w701) -> (element=w710:dbl)
              n504 = Less?(x=w705, y=w703) -> (x < y?=w704:bool)
              n505 = Less Or Equal To 0?(x=w710) -> (x <= 0?=w708:bool)
              n506 = And(x=w708, y=w704) -> (x .and. y?=w702:bool)
            }
            n507 = flat-sequence {
              tunnel: w613 -> [w679]
              tunnel: w609 -> [w678]
              tunnel: w612 -> [w677]
              tunnel: [w676] -> w610
              tunnel: w609 -> [w674]
              tunnel: w608 -> [w668]
              tunnel: w607 -> [w673]
              tunnel: w606 -> [w671]
              tunnel: w611 -> [w684]
              tunnel: w610 -> [w685]
              frame #0 {
                w670 = 0.06802721088435375  # AFR --> Lambda
                n508 = Multiply(x=w670, y=w668) -> (x*y=w669:dbl[])
                n509 = Select(t=w669, s=w671, f=w668) -> (s? t:f=w672:dbl[])
                n510 = control-ref of="Leistungs-Graph"() -> (w676:refnum<vi>)
                n511 = control-ref of="AFR,EGT-Graph"() -> (w675:refnum<vi>)
                n512 = call "UpdateGraph (SubVI).vi"("x"=w678, "Y2"=w679, "Y1"=w677, "XYGraph (Eingang)"=w676) -> ()  [unwired: 8 in]
                n513 = call "UpdateGraph (SubVI).vi"("x"=w674, "Y2"=w673, "Y1"=w672, "XYGraph (Eingang)"=w675) -> ()  [unwired: 8 in]
              }
              frame #1 {
                w680 = 1  # 0 = Keine Autoskalierung 1 = Autoskalierung
                w694 = 1
                w687 = 0
                n514 = Multiply(x=1.8, y=w684) -> (x*y=w693:dbl)
                n515 = property on="Eigenschaftsknoten" class="XYGraph (strikt)"(reference=w685, "ActYScl"=w687, "YScale.ScaleFit"=w694, "XScale.ScaleFit"=w694, "ActYScl"=w694, "YScale.Maximum"=w693, "YScale.Minimum"=w687) -> (reference out=w691:refnum<vi>)  [unwired: 1 in, 1 out]
                n516 = property on="Eigenschaftsknoten" class="XYGraph (strikt)"(reference=w691, "ActYScl"=w687) -> (reference out=w688:refnum<vi>, "YScale.Maximum"=w690:dbl, "XScale.Minimum"=w683:dbl, "XScale.Maximum"=w682:dbl)  [unwired: 1 in, 1 out]
                n517 = Add(x=w690, y=3.0) -> (x+y=w686:dbl)
                n518 = property on="Eigenschaftsknoten" class="XYGraph (strikt)"(reference=w688, "ActYScl"=w687, "YScale.Maximum"=w686) -> ()  [unwired: 1 in, 2 out]
                n519 = property on="AFR,EGT-Graph" class="XYGraph (strikt)"("XScale.Minimum"=w683, "XScale.Maximum"=w682, "ActYScl"=0, "YScale.ScaleFit"=w680, "ActYScl"=w680, "YScale.ScaleFit"=w680) -> ()  [unwired: 2 in, 2 out]
              }
            }
            n520 = local read "Übersetzung ermitteln aus"() -> (w605:T2)
            n521 = Increment(x=w656) -> (x+1=w614:i32)
            n522 = Array Subset "nWelle"(array=w630, index=w614) -> (w634:dbl[])  [unwired: 1 in]
            n523 = Array Subset "EGT"(array=w615, index=w614) -> (w607:dbl[])  [unwired: 1 in]
            n524 = Array Subset "AFR"(array=w616, index=w614) -> (w608:dbl[])  [unwired: 1 in]
            n525 = Array Max & Min "nWelle_max [1/min]"(array=w634) -> (max value=w636:dbl)  [unwired: 3 out]
            n526 = Array Subset "n"(array=w631, index=w614) -> (w654:dbl[])  [unwired: 1 in]
            n527 = Array Subset "M"(array=w632, index=w614) -> (w643:dbl[])  [unwired: 1 in]
            n528 = Array Max & Min "Mmax"(array=w643) -> (max value=w642:dbl, max index (indices)=w655:i32)  [unwired: 2 out]
            n529 = Array Max & Min "nmax [1/min]"(array=w654) -> (max value=w641:dbl)  [unwired: 3 out]
            n530 = Array Subset "P"(array=w633, index=w614) -> (w612:dbl[])  [unwired: 1 in]
            n531 = Index Array "n(Mmax)"(array=w654, index=w655) -> (element=w653:dbl)
            n532 = Array Max & Min "Pmax"(array=w612) -> (max value=w625:dbl, max index (indices)=w635:i32)  [unwired: 2 out]
            "Pmax" <- w625
            n533 = call "n2v (SubVI).vi"("Übersetzung ermitteln aus"=w605, "Array (Eingang)"=w654, "Rollenumfang [m]"=w644) -> ("Array (Ausgang)"=w609:dbl[], "Boolesch"=w646:bool)  [unwired: 7 in]
            n534 = Index Array "nWelle (Pmax)"(array=w634, index=w635) -> (element=w623:dbl)
            n535 = Index Array "n(Pmax)"(array=w654, index=w635) -> (element=w622:dbl)
            n536 = case shown="Standard" w605 {
              tunnel: [w697 w700] -> w613
              tunnel: w643 -> [w697 _]
              tunnel: w634 -> [_ w700]
              tunnel: w642 -> [w696 _]
              tunnel: [w696 w699] -> w611
              tunnel: w636 -> [_ w699]
              tunnel: [w695 w698] -> w624
              tunnel: w623 -> [_ w698]
              tunnel: w622 -> [w695 _]
              frame Default {
              }
              frame "vario (km/h)" {
              }
            }
            "n(Pmax)" <- w624
            n537 = Divide(x=w641, y=w650) -> (x/y=w663:dbl)
            n538 = local read "air temperature [°C]"() -> (w639:dbl)
            n539 = local read "air pressure [mbar]"() -> (w640:dbl)
            n540 = Format Into String(format string="%.1f PS" ("Format-String"), w625) -> (resulting string=→"Pmax":string)  [unwired: 2 in, 1 out]
            n541 = local read "Strecke [m]"() -> (w620:dbl)
            n542 = Compound Arithmetic op=MULTIPLY "v(Pmax)"(w622, w644, w645) -> (w651:dbl)
            n543 = Compound Arithmetic op=MULTIPLY "vmax"(w663, w644, w645) -> (w637:dbl)
            n544 = Format Date/Time String(time format string (%c)="%x %H:%M") -> (date/time string=w621:string)  [unwired: 2 in]
            "Datum+Zeit" <- w621
            n545 = Format Into String(format string="%.1f PS bei %d 1/min   |   %.1f Nm bei %d 1/min   |   vmax %d km/h\\nDIN 70020 k =%.3f (%d \\B0C, %d mbar)   |   %.0f m\\n%s" ("Format-String"), w625, w622, w642, w653, w637, w638, w639, w640, w620, w621) -> (resulting string=w649:string)  [unwired: 2 in, 1 out]
            n546 = Format Into String(format string="%.1f PS bei %d km/h, %d 1/min   |   vmax %d km/h\\nDIN 70020 k =%.3f (%d \\B0C, %d mbar)   |   %.0f m\\n%s" ("Format-String"), w625, w651, w623, w637, w638, w639, w640, w620, w621) -> (resulting string=w647:string)  [unwired: 2 in, 1 out]
            n547 = Select(t=w647, s=w646, f=w649) -> (s? t:f=→"Ergebnis":string)
            n548 = property on="Ergebnis" class="Str"("Text.FontSize"=18) -> ()  [unwired: 2 in, 2 out]
            n549 = property on="Pmax" class="Str"("Text.FontSize"=48) -> ()  [unwired: 2 in, 2 out]
          }
        }
        n550 = flat-sequence {
          tunnel: w401 -> [w552]
          tunnel: w365 -> [w545]
          tunnel: w366 -> [w546]
          tunnel: w402 -> [w553]
          tunnel: w403 -> [w547]
          tunnel: w404 -> [w554]
          tunnel: [w554] -> w425
          tunnel: [w547] -> w424
          tunnel: [w553] -> w423
          tunnel: [w546] -> w422
          tunnel: [w545] -> w421
          tunnel: [w552] -> w420
          tunnel: [w549] -> w390
          tunnel: w389 -> [w549]
          tunnel: [w548] -> w382
          tunnel: w381 -> [w548]
          tunnel: w361 -> [w544]
          tunnel: [w544] -> w364
          tunnel: w360 -> [w543]
          tunnel: [w543] -> w363
          tunnel: w349 -> [w539]
          tunnel: w348 -> [w538]
          tunnel: w425 -> [w599]
          tunnel: w424 -> [w598]
          tunnel: w423 -> [w597]
          tunnel: w422 -> [w596]
          tunnel: w421 -> [w595]
          tunnel: w420 -> [w594]
          tunnel: w390 -> [w579]
          tunnel: w382 -> [w576]
          tunnel: w364 -> [w562]
          tunnel: w363 -> [w561]
          frame #0 {
            w551 = FALSE ("Start [F1]")
            w542 = 0  # Aktivieren
            n551 = local write "Start"(w551) -> ()
            n552 = Not A Number/Path/Refnum?(number/path/refnum=w539) -> (NaN/Path/Refnum?=w541:bool)
            n553 = Not A Number/Path/Refnum?(number/path/refnum=w538) -> (NaN/Path/Refnum?=w540:bool)
            n554 = property on="Drucken" class="Bool. (strikt)"("DisabledEnum"=w542) -> ()  [unwired: 2 in, 2 out]
            n555 = property on="Übersetzung ermitteln aus" class="Enum (strikt)"("DisabledEnum"=w542) -> ()  [unwired: 2 in, 2 out]
            n556 = property on="Speichern" class="Bool. (strikt)"("DisabledEnum"=w542) -> ()  [unwired: 2 in, 2 out]
            n557 = property on="Konfiguration:" class="Bool. (strikt)"("DisabledEnum"=w542) -> ()  [unwired: 2 in, 2 out]
            n558 = property on="Ende" class="Bool. (strikt)"("DisabledEnum"=w542) -> ()  [unwired: 2 in, 2 out]
            n559 = property on="Logfiles" class="Bool. (strikt)"("DisabledEnum"=w542) -> ()  [unwired: 2 in, 2 out]
            n560 = property on="Untersetzung\nermittelt" class="Bool. (strikt)"("BoolText.Text"="GO" ("Boolescher Text.Text"), "Blinking"=w551) -> ()  [unwired: 2 in, 2 out]
            n561 = local write "Untersetzung\nermittelt"(w551) -> ()
            n562 = case shown="False" w541 {
              tunnel: w539 -> [w556 _]
              frame False {
                n563 = Close File(refnum=w556) -> ()  [unwired: 1 in, 2 out]
              }
              frame True {
              }
            }
            n564 = case shown="False" w540 {
              tunnel: w538 -> [w555 _]
              frame False {
                n565 = Close File(refnum=w555) -> ()  [unwired: 1 in, 2 out]
              }
              frame True {
              }
            }
          }
          frame #1 {
            # "Es können evtl. aus Datenspeicher noch mehrere Werte entfernt und für anderes verwendet \nwerden, da einige in diesem VI nicht beschrieben und evlt. auch in ReCalc nicht verwendet werden\n(ggf. in ReCalc prüfen ob das auch tatsächlich so ist)"
            n566 = local read "moving average Mittelwert"() -> (w588:u8)
            n567 = local read "air pressure [mbar]"() -> (w585:dbl)
            n568 = local read "Datum+Zeit"() -> (w568:string)
            n569 = local read "air temperature [°C]"() -> (w586:dbl)
            n570 = local read "difference quotient"() -> (w587:u8)
            n571 = local read "dynospeed of torque loss. n1 [1/min]"() -> (w575:u16)
            n572 = local read "Übersetzung ermitteln aus"() -> (w584:T2)
            n573 = local read "Title Diagram"() -> (w564:string)
            n574 = Path To String(path="Auto-Pfad") -> (string=w571:string)
            n575 = local read "tire circumferential  [m]"() -> (w589:dbl)
            n576 = local read "torque loss M0 [Nm] @ n = 0"() -> (w574:dbl)
            n577 = local read "torque loss M1 [Nm] @ n1"() -> (w573:dbl)
            n578 = local read "Messung Klimadaten"() -> (w581:bool)
            n579 = local read "Inertia dyno [kgm²]"() -> (w592:dbl)
            n580 = local read "ignition [Imp/rev]"() -> (w591:dbl)
            n581 = local read "n min [1/min]"() -> (w582:u16)
            n582 = local read "v min [km/h]"() -> (w577:u16)
            n583 = local read "nCrank/nDyno"() -> (w578:dbl)
            n584 = local read "gear ratio [1:]"() -> (w590:dbl)
            n585 = local read "AFR, EGT"() -> (w560:bool)
            n586 = Concatenate Strings(w568, "|", w571) -> (w570:string)
            n587 = local read "Lambda"() -> (w559:bool)
            n588 = local read "duration  [s]"() -> (w583:u8)
            n589 = local read "incr./rev. dyno  [Inkr/U]"() -> (w593:u16)
            n590 = Build Array(w560, w559) -> (w558:bool[])
            n591 = local read "Strecke [m]"() -> (w567:dbl)
            n592 = Boolean Array To Number(Boolean array=w558) -> (number=w557:u32)
            n593 = Concatenate Strings("Fahrzeugdaten", "§$", w564) -> (w566:string)
            n594 = Bundle(w566, w570, "incr./rev. dyno  [Inkr/U]"=w593, "circum. dyno [m]"=w596, "Inertia dyno [kgm²]"=w592, "ignition [Imp/rev]"=w591, "gear ratio [1:]"=w590, "tire circumferential  [m]"=w589, "mean value"=w597, "moving average Mittelwert"=w588, "difference quotient"=w587, w557, w599, "Strecke [m]"=w567, "air temperature [°C]"=w586, "dynospeed of torque loss. n1 [1/min]"=w575, "air pressure [mbar]"=w585, w598, w576, w562, w561, "Übersetzung ermitteln aus"=w584, "duration  [s]"=w583, "torque loss M0 [Nm] @ n = 0"=w574, "torque loss M1 [Nm] @ n1"=w573, "n min [1/min]"=w582, w595, w594, "Messung Klimadaten"=w581, "VISA-Referenz (Ausgang)"=w579, "nCrank/nDyno"=w578, "v min [km/h]"=w577) -> (→"Datenspeicher":T7)  [unwired: 1 in]
          }
          frame #2 {
            n595 = local read "Auto-Speichern"() -> (w602:bool)
            n596 = local read "Lauf abgebrochen"() -> (w601:bool)
            n597 = Not(x=w601) -> (.not. x?=w600:bool)
            n598 = And(x=w602, y=w600) -> (x .and. y?=w603:bool)
            n599 = case shown="True" w603 {
              frame False {
              }
              frame True {
                n600 = property on="Speichern" class="Bool. (strikt)"("Val(Sgnl)"=TRUE) -> ()  [unwired: 2 in, 2 out]
              }
            }
          }
        }
      }
    }
    n601 = Boolean To (0,1)(Boolean=w341) -> (0, 1=w342:i16)
    n602 = property on="Registerkarte 2" class="RKElem (strikt)"("Value"=w342) -> ()  [unwired: 2 in, 2 out]
    n603 = local read "Ende"() -> (w343:bool)
  }
  n604 = flat-sequence {
    tunnel: [w1172] -> w1
    tunnel: w1 -> [w1224]
    frame #0 {
      n605 = local read "Datenspeicher"() -> (w1193:T3)
      n606 = call <vilib>:"Application Directory.vi"() -> ("Application Directory"=w1215:path)
      n607 = Build Path(base path=w1215, name or relative path="Konfig.xml") -> (appended path=w1195:path)
      n608 = call "LoadCluster (SubVI).vi"("Datenspeicher"=w1193, "XML File Path"=w1195) -> ("Value"=w1194:T5)  [unwired: 7 in, 2 out]
      n609 = property on="Datenspeicher" class="Cluster (strikt)"("Value"=w1194) -> ()  [unwired: 2 in, 2 out]
      n610 = Unbundle(w1194) -> ("Fahrzeugdaten"=w1179:string, "Auto-Pfad"=w1187:string, "Rolle [Inkr/U]"=w1213:u16, "Rollenumfang [m]"=w1212:dbl, "Rollenträgheit [kgm²]"=w1211:dbl, "Zündung [Imp/U]"=w1210:dbl, "Getriebe [1:]"=w1209:dbl, "Reifenumfang [m]"=w1208:dbl, "element"=w1199:dbl, "Gl. Mittelwert"=w1207:u8, "Differenzenquotient"=w1206:u8, w1174:u8, "Lufttemperatur [°C]"=w1205:dbl, "Mv: n1 [1/min]"=w1189:dbl, "Luftdruck [mbar]"=w1204:dbl, "Übersetzung ermitteln aus"=w1201:u8, "[s]"=w1203:dbl, "Mv: M0 [Nm]"=w1191:dbl, "Mv: M1 [Nm]"=w1192:dbl, "n vom Gas [1/min]"=w1202:dbl, "Boolesch"=w1200:bool, "Serielle Schnittstelle"=w1198:refnum<visa-resource-name>, "nKuWe/nRolle"=w1197:dbl, "v vom Gas [km/h]"=w1196:dbl)  [unwired: 8 out]
      n611 = property on="duration  [s]" class="DigWert (strikt)"("Value"=w1203) -> ()  [unwired: 2 in, 2 out]
      n612 = property on="incr./rev. dyno  [Inkr/U]" class="DigWert (strikt)"("Value"=w1213) -> ()  [unwired: 2 in, 2 out]
      n613 = property on="circum. dyno [m]" class="DigWert (strikt)"("Value"=w1212) -> ()  [unwired: 2 in, 2 out]
      n614 = property on="Inertia dyno [kgm²]" class="DigWert (strikt)"("Value"=w1211) -> ()  [unwired: 2 in, 2 out]
      n615 = property on="ignition [Imp/rev]" class="DigWert (strikt)"("Value"=w1210) -> ()  [unwired: 2 in, 2 out]
      n616 = property on="gear ratio [1:]" class="DigWert (strikt)"("Value"=w1209) -> ()  [unwired: 2 in, 2 out]
      n617 = property on="tire circumferential  [m]" class="DigWert (strikt)"("Value"=w1208) -> ()  [unwired: 2 in, 2 out]
      n618 = property on="nCrank/nDyno" class="DigWert (strikt)"("Value"=w1199) -> ()  [unwired: 2 in, 2 out]
      n619 = property on="moving average Mittelwert" class="DigWert (strikt)"("Value"=w1207) -> ()  [unwired: 2 in, 2 out]
      n620 = property on="difference quotient" class="DigWert (strikt)"("Value"=w1206) -> ()  [unwired: 2 in, 2 out]
      n621 = property on="air temperature [°C]" class="DigWert (strikt)"("Value"=w1205) -> ()  [unwired: 2 in, 2 out]
      n622 = property on="air pressure [mbar]" class="DigWert (strikt)"("Value"=w1204) -> ()  [unwired: 2 in, 2 out]
      n623 = property on="Übersetzung ermitteln aus" class="Enum (strikt)"("Val(Sgnl)"=w1201) -> ()  [unwired: 2 in, 2 out]
      n624 = property on="n min [1/min]" class="DigWert (strikt)"("Value"=w1202) -> ()  [unwired: 2 in, 2 out]
      n625 = property on="Messung Klimadaten" class="Bool. (strikt)"("Val(Sgnl)"=w1200) -> ()  [unwired: 2 in, 2 out]
      n626 = local write "Serielle Schnittstelle"(w1198) -> ()
      n627 = property on="nCrank/nDyno" class="DigWert (strikt)"("Value"=w1197) -> ()  [unwired: 2 in, 2 out]
      n628 = property on="v min [km/h]" class="DigWert (strikt)"("Value"=w1196) -> ()  [unwired: 2 in, 2 out]
      n629 = Number To Boolean Array(number=w1174) -> (Boolean array=w1171:bool[])
      n630 = Index Array(array=w1171, index=0) -> (element=w1172:bool)
      n631 = Index Array(array=w1171, index=1) -> (element=w1169:bool)
      n632 = property on="torque loss M0 [Nm] @ n = 0" class="DigWert (strikt)"("Value"=w1191) -> ()  [unwired: 2 in, 2 out]
      n633 = property on="torque loss M1 [Nm] @ n1" class="DigWert (strikt)"("Value"=w1192) -> ()  [unwired: 2 in, 2 out]
      n634 = property on="Lambda" class="Bool. (strikt)"("Val(Sgnl)"=w1169) -> ()  [unwired: 2 in, 2 out]
      n635 = property on="AFR, EGT" class="Bool. (strikt)"("Value"=w1172) -> ()  [unwired: 2 in, 2 out]
      n636 = Max & Min(x=1, y=w1189) -> (max(x,y)=w1188:dbl)  [unwired: 1 out]
      n637 = Search/Split String "führendes Datum+Zeit wegschneiden"(string=w1187, search string/char (-)="|") -> (substring before match=w1182:string, match + rest of string=w1185:string)  [unwired: 1 in, 1 out]
      n638 = Search/Split String "führende Fahrzeugdaten wegschneiden"(string=w1179, search string/char (-)="§$") -> (substring before match=w1177:string, match + rest of string=w1178:string)  [unwired: 1 in, 1 out]
      n639 = property on="dynospeed of torque loss. n1 [1/min]" class="DigWert (strikt)"("Value"=w1188) -> ()  [unwired: 2 in, 2 out]
      n640 = String Subset(string=w1185, offset (0)=1) -> (substring=w1183:string)  [unwired: 1 in]
      n641 = String Subset(string=w1178, offset (0)=2) -> (substring=w1176:string)  [unwired: 1 in]
      n642 = String To Path(string=w1183) -> (path=w1175:path)
      n643 = property on="Fahrzeugdaten" class="Str"("Value"=w1177) -> ()  [unwired: 2 in, 2 out]
      n644 = property on="Title Diagram" class="Str"("Value"=w1176) -> ()  [unwired: 2 in, 2 out]
      n645 = property on="Auto-Pfad" class="Pfad"("Value"=w1175) -> ()  [unwired: 2 in, 2 out]
      n646 = property on="Datum+Zeit" class="Str"("Value"=w1182) -> ()  [unwired: 2 in, 2 out]
    }
    frame #1 {
      w1233 = 2  # Deaktivieren
      w1235 = 0.0  # Graphen löschen
      n647 = local read "Y-Koord. Graph-Reset-Button (782)"() -> (w1223:i32)
      n648 = local read "Serielle Schnittstelle"() -> (w1231:refnum<visa-resource-name>)
      n649 = local read "Höhe Leistungs-Graph (646)"() -> (w1225:u32)
      n650 = property on="Füllstand Lesepuffer" class="Schieber (strikt)"("Scale.Maximum"=100) -> ()  [unwired: 2 in, 2 out]
      n651 = property on="Frontpanel-Position" class="Bereich"("Origin"=T8 {"Horizontal"=8, "Vertical"=6}) -> ()  [unwired: 2 in, 2 out]
      n652 = control-ref of="Resetskalierung Leistung"() -> (w1221:refnum<vi>)
      n653 = property on="Drucken" class="Bool. (strikt)"("DisabledEnum"=w1233) -> ()  [unwired: 2 in, 2 out]
      n654 = property on="Speichern" class="Bool. (strikt)"("DisabledEnum"=w1233) -> ()  [unwired: 2 in, 2 out]
      n655 = Build Array(w1235) -> (w1234:dbl[])
      n656 = VISA Clear(VISA resource name=w1231) -> (VISA resource name out=w1230:refnum<visa-resource-name>, error out=w1229:errorcluster)  [unwired: 1 in]
      n657 = control-ref of="Autoskalierung Leistung"() -> (w1216:refnum<vi>)
      n658 = property on="Untersetzung-Graph" class="SVDiagr (strikt)"("History Data"=w1234) -> ()  [unwired: 2 in, 2 out]
      n659 = VISA Close(VISA resource name=w1230, error in (no error)=w1229) -> (error out=w1228:errorcluster)
      n660 = control-ref of="AFR,EGT-Graph"() -> (w1220:refnum<vi>)
      n661 = case shown="Kein Fehler" w1228 {
        tunnel: [T4."Enabled" ("Deaktiviert") T4."Disabled and Grayed Out" ("Deaktiviert")] -> w1227
        frame No Error {
        }
        frame Error {
        }
      }
      n662 = control-ref of="Leistungs-Graph"() -> (w1222:refnum<vi>)
      n663 = control-ref of="Lambda"() -> (w1217:refnum<vi>)
      n664 = control-ref of="AFR"() -> (w1219:refnum<vi>)
      n665 = control-ref of="[°C]"() -> (w1218:refnum<vi>)
      n666 = call "Enable_AFR_EGT_Graph (SubVI).vi"("Leistungsgraph"=w1222, "AFR EGT"=w1224, "Y-Koord. Graph-Reset-Button (782)"=w1223, "Lambda"=w1217, "Reset Skalierung"=w1221, "Höhe Leistungs-Graph"=w1225, "AFR EGT Gaph"=w1220, "Auto Skalierung"=w1216, "AFR"=w1219, "EGT [°C]"=w1218, "Skalierungsfaktor Leistungsgraph"=0.6666666666666666) -> ()  [unwired: 5 in]
      n667 = property on="Start" class="Bool. (strikt)"("DisabledEnum"=w1227) -> ()  [unwired: 2 in, 2 out]
    }
  }
  n668 = property on="Auto-Speichern" class="Bool. (strikt)"("Value"=w3) -> ()  [unwired: 2 in, 2 out]
  "Text Zündung" <- "Ignition"
  "Text Rolle" <- "Dyno"
  "Auto-Gespeichert" <- w3
  "Auto-Datei" <- ""
